vi "RLconnect.vi"() -> ()   [LabVIEW 2019]
uses:
  Ctrl/ublox-ui_main.ctl
  Ctrl/gnss_config-2.ctl
  Ctrl/Ntrip_Account_db.ctl
  Ctrl/Ntrip error-leds.ctl
  Ctrl/cmd_common.ctl
  Ctrl/cmd_ini-add-read.ctl
  Ctrl/cmd_ini-RW.ctl
  Ctrl/GNSS-Ntrip ref.ctl
  Gmap/gmap_fgv-cmd.ctl
  Ctrl/error_state-val.ctl
  Ctrl/GNSS-Ntrip config.ctl
  C:/Users/WeGo/Documents/GitHub/Ycar/LabVIEW/Gmap/dll/GMap.NET.WindowsForms.dll
  Gmap/dll/GMap.NET.WindowsForms.dll
panel:
  out "Error":T1={"GNSS Serial"=0, "NMEA val"=0, "Send Serial"=0, "Ntrip TCP"=0, "RTCM val"=0, "GMAP"=0, "TBD1"=2, "TBD2"=2, "TBD3"=2}
  in  "Send-Serial Start-Stop":bool
  in  "GNSS Start-Stop":bool
  in  "stop":bool
  in  "gmap center":bool
  in  "Gmap Lon":dbl format="%.7f"
  in  "Gmap Lat":dbl format="%.7f"
  in  "GMapControl":refnum<k24>(container)
  out "GNSS time":string
  out "Ntrip conn":bool
  out "NMEA val":bool
  in  "main tap":T2(tab)
  out "TM\nptn":u32(slide) scale=0.0..200.0
  out "Sea Level":dbl
  out "N of Satellites":i32
  out "TM graph":T3(graph)=[{"TM array"=[{"Y(E)"=195478.83340938148, "X(N)"=532749.6315443226}, {"Y(E)"=195478.83340938148, "X(N)"=532749.6315443226}, {"Y(E)"=195478.83340938148, "X(N)"=532749.6315443226}, {"Y(E)"=195478.83340938148, "X(N)"=532749.6315443226}, {"Y(E)"=195478.83340938148, "X(N)"=532749.6315443226}, {"Y(E)"=195478.83340938148, "X(N)"=532749.6315443226}, {"Y(E)"=195478.83340938148, "X(N)"=532749.6315443226}, {"Y(E)"=195478.83340938148, "X(N)"=532749.6315443226}, {"Y(E)"=195478.83340938148, "X(N)"=532749.6315443226}, {"Y(E)"=195478.83340938148, "X(N)"=532749.6315443226}, {"Y(E)"=195478.80387262133, "X(N)"=532749.5945652778}, {"Y(E)"=195478.80387262133, "X(N)"=532749.5945652778}, {"Y(E)"=195478.80387262133, "X(N)"=532749.5945652778}, {"Y(E)"=195478.80387262133, "X(N)"=532749.5945652778}, {"Y(E)"=195478.80387262133, "X(N)"=532749.5945652778}, {"Y(E)"=195478.80387262133, "X(N)"=532749.5945652778}, {"Y(E)"=195478.80387262133, "X(N)"=532749.5945652778}, {"Y(E)"=195478.80387262133, "X(N)"=532749.5945652778}, {"Y(E)"=195478.80387262133, "X(N)"=532749.5945652778}, {"Y(E)"=195478.80387262133, "X(N)"=532749.5945652778}, {"Y(E)"=195478.80387262133, "X(N)"=532749.5945652778}, {"Y(E)"=195478.80387262133, "X(N)"=532749.5945652778}, {"Y(E)"=195478.80387262133, "X(N)"=532749.5945652778}, {"Y(E)"=195478.86283602339, "X(N)"=532749.4650507653}, {"Y(E)"=195478.86283602339, "X(N)"=532749.4650507653}, {"Y(E)"=195478.86283602339, "X(N)"=532749.4650507653}, {"Y(E)"=195478.86283602339, "X(N)"=532749.4650507653}, {"Y(E)"=195478.86283602339, "X(N)"=532749.4650507653}, {"Y(E)"=195478.86283602339, "X(N)"=532749.4650507653}, {"Y(E)"=195478.86283602339, "X(N)"=532749.4650507653}, {"Y(E)"=195478.86283602339, "X(N)"=532749.4650507653}, {"Y(E)"=195478.86283602339, "X(N)"=532749.4650507653}, {"Y(E)"=195478.86283602339, "X(N)"=532749.4650507653}, {"Y(E)"=195478.86283602339, "X(N)"=532749.4650507653}, {"Y(E)"=195478.86283602339, "X(N)"=532749.4650507653}, {"Y(E)"=195478.86283602339, "X(N)"=532749.4650507653}, {"Y(E)"=195478.8185809412, "X(N)"=532749.5020697443}, {"Y(E)"=195478.8185809412, "X(N)"=532749.5020697443}, {"Y(E)"=195478.8185809412, "X(N)"=532749.5020697443}, {"Y(E)"=195478.8185809412, "X(N)"=532749.5020697443}, {"Y(E)"=195478.8185809412, "X(N)"=532749.5020697443}, {"Y(E)"=195478.8185809412, "X(N)"=532749.5020697443}, {"Y(E)"=195478.8185809412, "X(N)"=532749.5020697443}, {"Y(E)"=195478.8185809412, "X(N)"=532749.5020697443}, {"Y(E)"=195478.8185809412, "X(N)"=532749.5020697443}, {"Y(E)"=195478.8185809412, "X(N)"=532749.5020697443}, {"Y(E)"=195478.8185809412, "X(N)"=532749.5020697443}, {"Y(E)"=195478.8185809412, "X(N)"=532749.5020697443}, {"Y(E)"=195478.8185809412, "X(N)"=532749.5020697443}, {"Y(E)"=195478.8333493192, "X(N)"=532749.5205592669}, {"Y(E)"=195478.8333493192, "X(N)"=532749.5205592669}, {"Y(E)"=195478.8333493192, "X(N)"=532749.5205592669}, {"Y(E)"=195478.8333493192, "X(N)"=532749.5205592669}, {"Y(E)"=195478.8333493192, "X(N)"=532749.5205592669}, {"Y(E)"=195478.8333493192, "X(N)"=532749.5205592669}, {"Y(E)"=195478.8333493192, "X(N)"=532749.5205592669}, {"Y(E)"=195478.8333493192, "X(N)"=532749.5205592669}, {"Y(E)"=195478.8333493192, "X(N)"=532749.5205592669}, {"Y(E)"=195478.8333493192, "X(N)"=532749.5205592669}, {"Y(E)"=195478.8333493192, "X(N)"=532749.5205592669}, {"Y(E)"=195478.8333493192, "X(N)"=532749.5205592669}, {"Y(E)"=195478.81854089958, "X(N)"=532749.4280797082}, {"Y(E)"=195478.81854089958, "X(N)"=532749.4280797082}, {"Y(E)"=195478.81854089958, "X(N)"=532749.4280797082}, {"Y(E)"=195478.81854089958, "X(N)"=532749.4280797082}, {"Y(E)"=195478.81854089958, "X(N)"=532749.4280797082}, {"Y(E)"=195478.81854089958, "X(N)"=532749.4280797082}, {"Y(E)"=195478.81854089958, "X(N)"=532749.4280797082}, {"Y(E)"=195478.81854089958, "X(N)"=532749.4280797082}, {"Y(E)"=195478.81854089958, "X(N)"=532749.4280797082}, {"Y(E)"=195478.81854089958, "X(N)"=532749.4280797082}, {"Y(E)"=195478.81854089958, "X(N)"=532749.4280797082}, {"Y(E)"=195478.81854089958, "X(N)"=532749.4280797082}, {"Y(E)"=195478.81854089958, "X(N)"=532749.4280797082}, {"Y(E)"=195478.8332592258, "X(N)"=532749.3540816847}, {"Y(E)"=195478.8332592258, "X(N)"=532749.3540816847}, {"Y(E)"=195478.8332592258, "X(N)"=532749.3540816847}, {"Y(E)"=195478.8332592258, "X(N)"=532749.3540816847}, {"Y(E)"=195478.8332592258, "X(N)"=532749.3540816847}, {"Y(E)"=195478.8332592258, "X(N)"=532749.3540816847}, {"Y(E)"=195478.8332592258, "X(N)"=532749.3540816847}, {"Y(E)"=195478.8332592258, "X(N)"=532749.3540816847}, {"Y(E)"=195478.8332592258, "X(N)"=532749.3540816847}, {"Y(E)"=195478.8332592258, "X(N)"=532749.3540816847}, {"Y(E)"=195478.8332592258, "X(N)"=532749.3540816847}, {"Y(E)"=195478.8332592258, "X(N)"=532749.3540816847}, {"Y(E)"=195478.8332592258, "X(N)"=532749.3540816847}, {"Y(E)"=195478.61200383154, "X(N)"=532749.5761715989}, {"Y(E)"=195478.61200383154, "X(N)"=532749.5761715989}, {"Y(E)"=195478.61200383154, "X(N)"=532749.5761715989}, {"Y(E)"=195478.61200383154, "X(N)"=532749.5761715989}, {"Y(E)"=195478.61200383154, "X(N)"=532749.5761715989}, {"Y(E)"=195478.61200383154, "X(N)"=532749.5761715989}, {"Y(E)"=195478.61200383154, "X(N)"=532749.5761715989}, {"Y(E)"=195478.61200383154, "X(N)"=532749.5761715989}, {"Y(E)"=195478.61200383154, "X(N)"=532749.5761715989}, {"Y(E)"=195478.61200383154, "X(N)"=532749.5761715989}, {"Y(E)"=195478.61200383154, "X(N)"=532749.5761715989}, {"Y(E)"=195478.61200383154, "X(N)"=532749.5761715989}, {"Y(E)"=195478.61200383154, "X(N)"=532749.5761715989}, {"Y(E)"=195478.61197379892, "X(N)"=532749.5206790727}, {"Y(E)"=195478.61197379892, "X(N)"=532749.5206790727}, {"Y(E)"=195478.61197379892, "X(N)"=532749.5206790727}, {"Y(E)"=195478.61197379892, "X(N)"=532749.5206790727}, {"Y(E)"=195478.61197379892, "X(N)"=532749.5206790727}, {"Y(E)"=195478.61197379892, "X(N)"=532749.5206790727}, {"Y(E)"=195478.61197379892, "X(N)"=532749.5206790727}, {"Y(E)"=195478.61197379892, "X(N)"=532749.5206790727}, {"Y(E)"=195478.61197379892, "X(N)"=532749.5206790727}, {"Y(E)"=195478.61197379892, "X(N)"=532749.5206790727}, {"Y(E)"=195478.61197379892, "X(N)"=532749.5206790727}, {"Y(E)"=195478.61197379892, "X(N)"=532749.5206790727}, {"Y(E)"=195478.61197379892, "X(N)"=532749.5206790727}, {"Y(E)"=195478.64144048005, "X(N)"=532749.4281755526}, {"Y(E)"=195478.64144048005, "X(N)"=532749.4281755526}, {"Y(E)"=195478.64144048005, "X(N)"=532749.4281755526}, {"Y(E)"=195478.64144048005, "X(N)"=532749.4281755526}, {"Y(E)"=195478.64144048005, "X(N)"=532749.4281755526}, {"Y(E)"=195478.64144048005, "X(N)"=532749.4281755526}, {"Y(E)"=195478.64144048005, "X(N)"=532749.4281755526}, {"Y(E)"=195478.64144048005, "X(N)"=532749.4281755526}, {"Y(E)"=195478.64144048005, "X(N)"=532749.4281755526}, {"Y(E)"=195478.64144048005, "X(N)"=532749.4281755526}, {"Y(E)"=195478.64144048005, "X(N)"=532749.4281755526}, {"Y(E)"=195478.64144048005, "X(N)"=532749.4281755526}, {"Y(E)"=195478.64144048005, "X(N)"=532749.4281755526}, {"Y(E)"=195478.56754852948, "X(N)"=532749.2432403986}, {"Y(E)"=195478.56754852948, "X(N)"=532749.2432403986}, {"Y(E)"=195478.56754852948, "X(N)"=532749.2432403986}, {"Y(E)"=195478.56754852948, "X(N)"=532749.2432403986}, {"Y(E)"=195478.56754852948, "X(N)"=532749.2432403986}, {"Y(E)"=195478.56754852948, "X(N)"=532749.2432403986}, {"Y(E)"=195478.56754852948, "X(N)"=532749.2432403986}, {"Y(E)"=195478.56754852948, "X(N)"=532749.2432403986}, {"Y(E)"=195478.56754852948, "X(N)"=532749.2432403986}, {"Y(E)"=195478.56754852948, "X(N)"=532749.2432403986}, {"Y(E)"=195478.56754852948, "X(N)"=532749.2432403986}, {"Y(E)"=195478.56754852948, "X(N)"=532749.2432403986}, {"Y(E)"=195478.56754852948, "X(N)"=532749.2432403986}, {"Y(E)"=195478.5822568451, "X(N)"=532749.1507448669}, {"Y(E)"=195478.5822568451, "X(N)"=532749.1507448669}, {"Y(E)"=195478.5822568451, "X(N)"=532749.1507448669}, {"Y(E)"=195478.5822568451, "X(N)"=532749.1507448669}, {"Y(E)"=195478.5822568451, "X(N)"=532749.1507448669}, {"Y(E)"=195478.5822568451, "X(N)"=532749.1507448669}, {"Y(E)"=195478.5822568451, "X(N)"=532749.1507448669}, {"Y(E)"=195478.5822568451, "X(N)"=532749.1507448669}, {"Y(E)"=195478.5822568451, "X(N)"=532749.1507448669}, {"Y(E)"=195478.5822568451, "X(N)"=532749.1507448669}, {"Y(E)"=195478.5822568451, "X(N)"=532749.1507448669}, {"Y(E)"=195478.5822568451, "X(N)"=532749.1507448669}, {"Y(E)"=195478.5822568451, "X(N)"=532749.1507448669}, {"Y(E)"=195478.3755095352, "X(N)"=532748.9103890732}, {"Y(E)"=195478.3755095352, "X(N)"=532748.9103890732}, {"Y(E)"=195478.3755095352, "X(N)"=532748.9103890732}, {"Y(E)"=195478.3755095352, "X(N)"=532748.9103890732}, {"Y(E)"=195478.3755095352, "X(N)"=532748.9103890732}, {"Y(E)"=195478.3755095352, "X(N)"=532748.9103890732}, {"Y(E)"=195478.3755095352, "X(N)"=532748.9103890732}, {"Y(E)"=195478.3755095352, "X(N)"=532748.9103890732}, {"Y(E)"=195478.3755095352, "X(N)"=532748.9103890732}, {"Y(E)"=195478.3755095352, "X(N)"=532748.9103890732}, {"Y(E)"=195478.3755095352, "X(N)"=532748.9103890732}, {"Y(E)"=195478.3755095352, "X(N)"=532748.9103890732}, {"Y(E)"=195478.3755095352, "X(N)"=532748.9103890732}, {"Y(E)"=195478.37543945547, "X(N)"=532748.78090651}, {"Y(E)"=195478.37543945547, "X(N)"=532748.78090651}, {"Y(E)"=195478.37543945547, "X(N)"=532748.78090651}, {"Y(E)"=195478.37543945547, "X(N)"=532748.78090651}, {"Y(E)"=195478.37543945547, "X(N)"=532748.78090651}, {"Y(E)"=195478.37543945547, "X(N)"=532748.78090651}, {"Y(E)"=195478.37543945547, "X(N)"=532748.78090651}, {"Y(E)"=195478.37543945547, "X(N)"=532748.78090651}, {"Y(E)"=195478.37543945547, "X(N)"=532748.78090651}, {"Y(E)"=195478.37543945547, "X(N)"=532748.78090651}, {"Y(E)"=195478.37543945547, "X(N)"=532748.78090651}, {"Y(E)"=195478.37543945547, "X(N)"=532748.78090651}, {"Y(E)"=195478.5082848043, "X(N)"=532748.8178296402}, {"Y(E)"=195478.5082848043, "X(N)"=532748.8178296402}, {"Y(E)"=195478.5082848043, "X(N)"=532748.8178296402}, {"Y(E)"=195478.5082848043, "X(N)"=532748.8178296402}, {"Y(E)"=195478.5082848043, "X(N)"=532748.8178296402}, {"Y(E)"=195478.5082848043, "X(N)"=532748.8178296402}, {"Y(E)"=195478.5082848043, "X(N)"=532748.8178296402}, {"Y(E)"=195478.5082848043, "X(N)"=532748.8178296402}, {"Y(E)"=195478.5082848043, "X(N)"=532748.8178296402}, {"Y(E)"=195478.5082848043, "X(N)"=532748.8178296402}, {"Y(E)"=195478.5082848043, "X(N)"=532748.8178296402}, {"Y(E)"=195478.5082848043, "X(N)"=532748.8178296402}, {"Y(E)"=195478.5082848043, "X(N)"=532748.8178296402}, {"Y(E)"=195478.7001636224, "X(N)"=532748.8547208244}, {"Y(E)"=195478.7001636224, "X(N)"=532748.8547208244}, {"Y(E)"=195478.7001636224, "X(N)"=532748.8547208244}, {"Y(E)"=195478.7001636224, "X(N)"=532748.8547208244}, {"Y(E)"=195478.7001636224, "X(N)"=532748.8547208244}, {"Y(E)"=195478.7001636224, "X(N)"=532748.8547208244}, {"Y(E)"=195478.7001636224, "X(N)"=532748.8547208244}, {"Y(E)"=195478.7001636224, "X(N)"=532748.8547208244}, {"Y(E)"=195478.7001636224, "X(N)"=532748.8547208244}, {"Y(E)"=195478.7001636224, "X(N)"=532748.8547208244}]}, {"TM array"=[{"Y(E)"=195478.60442441847, "X(N)"=532749.6892681528}, {"Y(E)"=195478.63475492285, "X(N)"=532749.6883149784}, {"Y(E)"=195478.6649657266, "X(N)"=532749.6854592166}, {"Y(E)"=195478.69493760145, "X(N)"=532749.680712138}, {"Y(E)"=195478.72455226214, "X(N)"=532749.6740924771}, {"Y(E)"=195478.7536928331, "X(N)"=532749.6656263586}, {"Y(E)"=195478.7822443098, "X(N)"=532749.6553471944}, {"Y(E)"=195478.81009401265, "X(N)"=532749.6432955518}, {"Y(E)"=195478.83713203156, "X(N)"=532749.6295189931}, {"Y(E)"=195478.86325165984, "X(N)"=532749.6140718879}, {"Y(E)"=195478.88834981524, "X(N)"=532749.5970151991}, {"Y(E)"=195478.91232744683, "X(N)"=532749.5784162417}, {"Y(E)"=195478.93508992583, "X(N)"=532749.5583484169}, {"Y(E)"=195478.95654741913, "X(N)"=532749.5368909236}, {"Y(E)"=195478.97661524382, "X(N)"=532749.5141284446}, {"Y(E)"=195478.99521420136, "X(N)"=532749.490150813}, {"Y(E)"=195479.01227089018, "X(N)"=532749.4650526576}, {"Y(E)"=195479.02771799528, "X(N)"=532749.4389330294}, {"Y(E)"=195479.04149455403, "X(N)"=532749.4118950105}, {"Y(E)"=195479.0535461966, "X(N)"=532749.3840453076}, {"Y(E)"=195479.06382536073, "X(N)"=532749.3554938309}, {"Y(E)"=195479.0722914792, "X(N)"=532749.32635326}, {"Y(E)"=195479.07891114015, "X(N)"=532749.2967385993}, {"Y(E)"=195479.0836582188, "X(N)"=532749.2667667244}, {"Y(E)"=195479.08651398055, "X(N)"=532749.2365559207}, {"Y(E)"=195479.08746715504, "X(N)"=532749.2062254163}, {"Y(E)"=195479.08651398055, "X(N)"=532749.1758949119}, {"Y(E)"=195479.0836582188, "X(N)"=532749.1456841081}, {"Y(E)"=195479.07891114015, "X(N)"=532749.1157122332}, {"Y(E)"=195479.0722914792, "X(N)"=532749.0860975726}, {"Y(E)"=195479.06382536073, "X(N)"=532749.0569570017}, {"Y(E)"=195479.0535461966, "X(N)"=532749.0284055249}, {"Y(E)"=195479.04149455403, "X(N)"=532749.000555822}, {"Y(E)"=195479.02771799528, "X(N)"=532748.9735178031}, {"Y(E)"=195479.01227089018, "X(N)"=532748.9473981749}, {"Y(E)"=195478.99521420136, "X(N)"=532748.9223000195}, {"Y(E)"=195478.97661524382, "X(N)"=532748.898322388}, {"Y(E)"=195478.95654741913, "X(N)"=532748.8755599089}, {"Y(E)"=195478.93508992583, "X(N)"=532748.8541024156}, {"Y(E)"=195478.91232744683, "X(N)"=532748.8340345909}, {"Y(E)"=195478.88834981524, "X(N)"=532748.8154356334}, {"Y(E)"=195478.86325165984, "X(N)"=532748.7983789446}, {"Y(E)"=195478.83713203156, "X(N)"=532748.7829318395}, {"Y(E)"=195478.81009401265, "X(N)"=532748.7691552808}, {"Y(E)"=195478.7822443098, "X(N)"=532748.7571036381}, {"Y(E)"=195478.7536928331, "X(N)"=532748.746824474}, {"Y(E)"=195478.72455226214, "X(N)"=532748.7383583555}, {"Y(E)"=195478.69493760145, "X(N)"=532748.7317386946}, {"Y(E)"=195478.6649657266, "X(N)"=532748.726991616}, {"Y(E)"=195478.63475492285, "X(N)"=532748.7241358542}, {"Y(E)"=195478.60442441847, "X(N)"=532748.7231826797}, {"Y(E)"=195478.5740939141, "X(N)"=532748.7241358542}, {"Y(E)"=195478.54388311034, "X(N)"=532748.726991616}, {"Y(E)"=195478.5139112355, "X(N)"=532748.7317386946}, {"Y(E)"=195478.4842965748, "X(N)"=532748.7383583555}, {"Y(E)"=195478.45515600385, "X(N)"=532748.746824474}, {"Y(E)"=195478.42660452714, "X(N)"=532748.7571036381}, {"Y(E)"=195478.3987548243, "X(N)"=532748.7691552808}, {"Y(E)"=195478.37171680538, "X(N)"=532748.7829318395}, {"Y(E)"=195478.3455971771, "X(N)"=532748.7983789446}, {"Y(E)"=195478.3204990217, "X(N)"=532748.8154356334}, {"Y(E)"=195478.29652139012, "X(N)"=532748.8340345909}, {"Y(E)"=195478.27375891112, "X(N)"=532748.8541024156}, {"Y(E)"=195478.25230141782, "X(N)"=532748.8755599089}, {"Y(E)"=195478.23223359312, "X(N)"=532748.898322388}, {"Y(E)"=195478.21363463558, "X(N)"=532748.9223000195}, {"Y(E)"=195478.19657794677, "X(N)"=532748.9473981749}, {"Y(E)"=195478.18113084167, "X(N)"=532748.9735178031}, {"Y(E)"=195478.16735428292, "X(N)"=532749.000555822}, {"Y(E)"=195478.15530264034, "X(N)"=532749.0284055249}, {"Y(E)"=195478.14502347622, "X(N)"=532749.0569570017}, {"Y(E)"=195478.13655735774, "X(N)"=532749.0860975726}, {"Y(E)"=195478.1299376968, "X(N)"=532749.1157122332}, {"Y(E)"=195478.12519061816, "X(N)"=532749.1456841081}, {"Y(E)"=195478.1223348564, "X(N)"=532749.1758949119}, {"Y(E)"=195478.1213816819, "X(N)"=532749.2062254163}, {"Y(E)"=195478.1223348564, "X(N)"=532749.2365559207}, {"Y(E)"=195478.12519061816, "X(N)"=532749.2667667244}, {"Y(E)"=195478.1299376968, "X(N)"=532749.2967385993}, {"Y(E)"=195478.13655735774, "X(N)"=532749.32635326}, {"Y(E)"=195478.14502347622, "X(N)"=532749.3554938309}, {"Y(E)"=195478.15530264034, "X(N)"=532749.3840453076}, {"Y(E)"=195478.16735428292, "X(N)"=532749.4118950105}, {"Y(E)"=195478.18113084167, "X(N)"=532749.4389330294}, {"Y(E)"=195478.19657794677, "X(N)"=532749.4650526576}, {"Y(E)"=195478.21363463558, "X(N)"=532749.490150813}, {"Y(E)"=195478.23223359312, "X(N)"=532749.5141284446}, {"Y(E)"=195478.25230141782, "X(N)"=532749.5368909236}, {"Y(E)"=195478.27375891112, "X(N)"=532749.5583484169}, {"Y(E)"=195478.29652139012, "X(N)"=532749.5784162417}, {"Y(E)"=195478.3204990217, "X(N)"=532749.5970151991}, {"Y(E)"=195478.3455971771, "X(N)"=532749.6140718879}, {"Y(E)"=195478.37171680538, "X(N)"=532749.6295189931}, {"Y(E)"=195478.3987548243, "X(N)"=532749.6432955518}, {"Y(E)"=195478.42660452714, "X(N)"=532749.6553471944}, {"Y(E)"=195478.45515600385, "X(N)"=532749.6656263586}, {"Y(E)"=195478.4842965748, "X(N)"=532749.6740924771}, {"Y(E)"=195478.5139112355, "X(N)"=532749.680712138}, {"Y(E)"=195478.54388311034, "X(N)"=532749.6854592166}, {"Y(E)"=195478.5740939141, "X(N)"=532749.6883149784}, {"Y(E)"=195478.60442441847, "X(N)"=532749.6892681528}]}, {"TM array"=[{"Y(E)"=195478.60442441847, "X(N)"=532750.2062254163}, {"Y(E)"=195478.667214938, "X(N)"=532750.2042521447}, {"Y(E)"=195478.72975765204, "X(N)"=532750.1983401176}, {"Y(E)"=195478.79180573305, "X(N)"=532750.188512667}, {"Y(E)"=195478.85311430565, "X(N)"=532750.1748085774}, {"Y(E)"=195478.91344141285, "X(N)"=532750.1572819325}, {"Y(E)"=195478.97254897116, "X(N)"=532750.1360019022}, {"Y(E)"=195479.03020371005, "X(N)"=532750.1110524688}, {"Y(E)"=195479.08617809258, "X(N)"=532750.0825320963}, {"Y(E)"=195479.14025121345, "X(N)"=532750.0505533417}, {"Y(E)"=195479.19220967076, "X(N)"=532750.0152424106}, {"Y(E)"=195479.24184840822, "X(N)"=532749.9767386591}, {"Y(E)"=195479.2889715244, "X(N)"=532749.9351940437}, {"Y(E)"=195479.3333930459, "X(N)"=532749.8907725222}, {"Y(E)"=195479.37493766125, "X(N)"=532749.843649406}, {"Y(E)"=195479.41344141285, "X(N)"=532749.7940106685}, {"Y(E)"=195479.44875234397, "X(N)"=532749.7420522113}, {"Y(E)"=195479.4807310985, "X(N)"=532749.6879790904}, {"Y(E)"=195479.50925147094, "X(N)"=532749.6320047078}, {"Y(E)"=195479.53420090437, "X(N)"=532749.5743499689}, {"Y(E)"=195479.55548093477, "X(N)"=532749.5152424106}, {"Y(E)"=195479.5730075796, "X(N)"=532749.4549153034}, {"Y(E)"=195479.5867116692, "X(N)"=532749.3936067309}, {"Y(E)"=195479.59653911978, "X(N)"=532749.3315586499}, {"Y(E)"=195479.6024511469, "X(N)"=532749.2690159358}, {"Y(E)"=195479.60442441847, "X(N)"=532749.2062254163}, {"Y(E)"=195479.6024511469, "X(N)"=532749.1434348967}, {"Y(E)"=195479.59653911978, "X(N)"=532749.0808921827}, {"Y(E)"=195479.5867116692, "X(N)"=532749.0188441017}, {"Y(E)"=195479.5730075796, "X(N)"=532748.9575355292}, {"Y(E)"=195479.55548093477, "X(N)"=532748.897208422}, {"Y(E)"=195479.53420090437, "X(N)"=532748.8381008636}, {"Y(E)"=195479.50925147094, "X(N)"=532748.7804461247}, {"Y(E)"=195479.4807310985, "X(N)"=532748.7244717422}, {"Y(E)"=195479.44875234397, "X(N)"=532748.6703986212}, {"Y(E)"=195479.41344141285, "X(N)"=532748.618440164}, {"Y(E)"=195479.37493766125, "X(N)"=532748.5688014266}, {"Y(E)"=195479.3333930459, "X(N)"=532748.5216783104}, {"Y(E)"=195479.2889715244, "X(N)"=532748.4772567889}, {"Y(E)"=195479.24184840822, "X(N)"=532748.4357121735}, {"Y(E)"=195479.19220967076, "X(N)"=532748.397208422}, {"Y(E)"=195479.14025121345, "X(N)"=532748.3618974908}, {"Y(E)"=195479.08617809258, "X(N)"=532748.3299187362}, {"Y(E)"=195479.03020371005, "X(N)"=532748.3013983638}, {"Y(E)"=195478.97254897116, "X(N)"=532748.2764489304}, {"Y(E)"=195478.91344141285, "X(N)"=532748.2551689}, {"Y(E)"=195478.85311430565, "X(N)"=532748.2376422551}, {"Y(E)"=195478.79180573305, "X(N)"=532748.2239381656}, {"Y(E)"=195478.72975765204, "X(N)"=532748.214110715}, {"Y(E)"=195478.667214938, "X(N)"=532748.2081986879}, {"Y(E)"=195478.60442441847, "X(N)"=532748.2062254163}, {"Y(E)"=195478.54163389895, "X(N)"=532748.2081986879}, {"Y(E)"=195478.4790911849, "X(N)"=532748.214110715}, {"Y(E)"=195478.4170431039, "X(N)"=532748.2239381656}, {"Y(E)"=195478.3557345313, "X(N)"=532748.2376422551}, {"Y(E)"=195478.2954074241, "X(N)"=532748.2551689}, {"Y(E)"=195478.2362998658, "X(N)"=532748.2764489304}, {"Y(E)"=195478.1786451269, "X(N)"=532748.3013983638}, {"Y(E)"=195478.12267074437, "X(N)"=532748.3299187362}, {"Y(E)"=195478.0685976235, "X(N)"=532748.3618974908}, {"Y(E)"=195478.0166391662, "X(N)"=532748.397208422}, {"Y(E)"=195477.96700042873, "X(N)"=532748.4357121735}, {"Y(E)"=195477.91987731255, "X(N)"=532748.4772567889}, {"Y(E)"=195477.87545579104, "X(N)"=532748.5216783104}, {"Y(E)"=195477.8339111757, "X(N)"=532748.5688014266}, {"Y(E)"=195477.7954074241, "X(N)"=532748.618440164}, {"Y(E)"=195477.76009649297, "X(N)"=532748.6703986212}, {"Y(E)"=195477.72811773844, "X(N)"=532748.7244717422}, {"Y(E)"=195477.699597366, "X(N)"=532748.7804461247}, {"Y(E)"=195477.67464793258, "X(N)"=532748.8381008636}, {"Y(E)"=195477.65336790218, "X(N)"=532748.897208422}, {"Y(E)"=195477.63584125735, "X(N)"=532748.9575355292}, {"Y(E)"=195477.62213716775, "X(N)"=532749.0188441017}, {"Y(E)"=195477.61230971717, "X(N)"=532749.0808921827}, {"Y(E)"=195477.60639769005, "X(N)"=532749.1434348967}, {"Y(E)"=195477.60442441847, "X(N)"=532749.2062254163}, {"Y(E)"=195477.60639769005, "X(N)"=532749.2690159358}, {"Y(E)"=195477.61230971717, "X(N)"=532749.3315586499}, {"Y(E)"=195477.62213716775, "X(N)"=532749.3936067309}, {"Y(E)"=195477.63584125735, "X(N)"=532749.4549153034}, {"Y(E)"=195477.65336790218, "X(N)"=532749.5152424106}, {"Y(E)"=195477.67464793258, "X(N)"=532749.5743499689}, {"Y(E)"=195477.699597366, "X(N)"=532749.6320047078}, {"Y(E)"=195477.72811773844, "X(N)"=532749.6879790904}, {"Y(E)"=195477.76009649297, "X(N)"=532749.7420522113}, {"Y(E)"=195477.7954074241, "X(N)"=532749.7940106685}, {"Y(E)"=195477.8339111757, "X(N)"=532749.843649406}, {"Y(E)"=195477.87545579104, "X(N)"=532749.8907725222}, {"Y(E)"=195477.91987731255, "X(N)"=532749.9351940437}, {"Y(E)"=195477.96700042873, "X(N)"=532749.9767386591}, {"Y(E)"=195478.0166391662, "X(N)"=532750.0152424106}, {"Y(E)"=195478.0685976235, "X(N)"=532750.0505533417}, {"Y(E)"=195478.12267074437, "X(N)"=532750.0825320963}, {"Y(E)"=195478.1786451269, "X(N)"=532750.1110524688}, {"Y(E)"=195478.2362998658, "X(N)"=532750.1360019022}, {"Y(E)"=195478.2954074241, "X(N)"=532750.1572819325}, {"Y(E)"=195478.3557345313, "X(N)"=532750.1748085774}, {"Y(E)"=195478.4170431039, "X(N)"=532750.188512667}, {"Y(E)"=195478.4790911849, "X(N)"=532750.1983401176}, {"Y(E)"=195478.54163389895, "X(N)"=532750.2042521447}, {"Y(E)"=195478.60442441847, "X(N)"=532750.2062254163}]}, {"TM array"=[{"Y(E)"=195478.60442441847, "X(N)"=532751.2062254163}, {"Y(E)"=195478.73000545753, "X(N)"=532751.2022788732}, {"Y(E)"=195478.8550908856, "X(N)"=532751.1904548189}, {"Y(E)"=195478.97918704763, "X(N)"=532751.1707999178}, {"Y(E)"=195479.10180419282, "X(N)"=532751.1433917385}, {"Y(E)"=195479.22245840722, "X(N)"=532751.1083384489}, {"Y(E)"=195479.34067352384, "X(N)"=532751.0657783881}, {"Y(E)"=195479.4559830016, "X(N)"=532751.0158795213}, {"Y(E)"=195479.56793176668, "X(N)"=532750.9588387763}, {"Y(E)"=195479.67607800843, "X(N)"=532750.8948812673}, {"Y(E)"=195479.77999492307, "X(N)"=532750.824259405}, {"Y(E)"=195479.879272398, "X(N)"=532750.7472519018}, {"Y(E)"=195479.97351863034, "X(N)"=532750.6641626711}, {"Y(E)"=195480.0623616733, "X(N)"=532750.5753196281}, {"Y(E)"=195480.14545090403, "X(N)"=532750.4810733958}, {"Y(E)"=195480.22245840722, "X(N)"=532750.3817959209}, {"Y(E)"=195480.29308026948, "X(N)"=532750.2778790062}, {"Y(E)"=195480.35703777857, "X(N)"=532750.1697327645}, {"Y(E)"=195480.4140785234, "X(N)"=532750.0577839994}, {"Y(E)"=195480.46397739026, "X(N)"=532749.9424745217}, {"Y(E)"=195480.50653745106, "X(N)"=532749.824259405}, {"Y(E)"=195480.54159074073, "X(N)"=532749.7036051906}, {"Y(E)"=195480.56899891995, "X(N)"=532749.5809880454}, {"Y(E)"=195480.5886538211, "X(N)"=532749.4568918834}, {"Y(E)"=195480.60047787533, "X(N)"=532749.3318064554}, {"Y(E)"=195480.60442441847, "X(N)"=532749.2062254163}, {"Y(E)"=195480.60047787533, "X(N)"=532749.0806443772}, {"Y(E)"=195480.5886538211, "X(N)"=532748.9555589492}, {"Y(E)"=195480.56899891995, "X(N)"=532748.8314627871}, {"Y(E)"=195480.54159074073, "X(N)"=532748.7088456419}, {"Y(E)"=195480.50653745106, "X(N)"=532748.5881914275}, {"Y(E)"=195480.46397739026, "X(N)"=532748.4699763109}, {"Y(E)"=195480.4140785234, "X(N)"=532748.3546668332}, {"Y(E)"=195480.35703777857, "X(N)"=532748.2427180681}, {"Y(E)"=195480.29308026948, "X(N)"=532748.1345718263}, {"Y(E)"=195480.22245840722, "X(N)"=532748.0306549117}, {"Y(E)"=195480.14545090403, "X(N)"=532747.9313774367}, {"Y(E)"=195480.0623616733, "X(N)"=532747.8371312044}, {"Y(E)"=195479.97351863034, "X(N)"=532747.7482881615}, {"Y(E)"=195479.879272398, "X(N)"=532747.6651989308}, {"Y(E)"=195479.77999492307, "X(N)"=532747.5881914275}, {"Y(E)"=195479.67607800843, "X(N)"=532747.5175695652}, {"Y(E)"=195479.56793176668, "X(N)"=532747.4536120562}, {"Y(E)"=195479.4559830016, "X(N)"=532747.3965713113}, {"Y(E)"=195479.34067352384, "X(N)"=532747.3466724445}, {"Y(E)"=195479.22245840722, "X(N)"=532747.3041123836}, {"Y(E)"=195479.10180419282, "X(N)"=532747.269059094}, {"Y(E)"=195478.97918704763, "X(N)"=532747.2416509148}, {"Y(E)"=195478.8550908856, "X(N)"=532747.2219960137}, {"Y(E)"=195478.73000545753, "X(N)"=532747.2101719594}, {"Y(E)"=195478.60442441847, "X(N)"=532747.2062254163}, {"Y(E)"=195478.47884337942, "X(N)"=532747.2101719594}, {"Y(E)"=195478.35375795135, "X(N)"=532747.2219960137}, {"Y(E)"=195478.22966178932, "X(N)"=532747.2416509148}, {"Y(E)"=195478.10704464413, "X(N)"=532747.269059094}, {"Y(E)"=195477.98639042972, "X(N)"=532747.3041123836}, {"Y(E)"=195477.8681753131, "X(N)"=532747.3466724445}, {"Y(E)"=195477.75286583535, "X(N)"=532747.3965713113}, {"Y(E)"=195477.64091707027, "X(N)"=532747.4536120562}, {"Y(E)"=195477.53277082852, "X(N)"=532747.5175695652}, {"Y(E)"=195477.42885391388, "X(N)"=532747.5881914275}, {"Y(E)"=195477.32957643896, "X(N)"=532747.6651989308}, {"Y(E)"=195477.2353302066, "X(N)"=532747.7482881615}, {"Y(E)"=195477.14648716364, "X(N)"=532747.8371312044}, {"Y(E)"=195477.0633979329, "X(N)"=532747.9313774367}, {"Y(E)"=195476.98639042972, "X(N)"=532748.0306549117}, {"Y(E)"=195476.91576856747, "X(N)"=532748.1345718263}, {"Y(E)"=195476.85181105838, "X(N)"=532748.2427180681}, {"Y(E)"=195476.79477031354, "X(N)"=532748.3546668332}, {"Y(E)"=195476.7448714467, "X(N)"=532748.4699763109}, {"Y(E)"=195476.7023113859, "X(N)"=532748.5881914275}, {"Y(E)"=195476.66725809622, "X(N)"=532748.7088456419}, {"Y(E)"=195476.639849917, "X(N)"=532748.8314627871}, {"Y(E)"=195476.62019501586, "X(N)"=532748.9555589492}, {"Y(E)"=195476.60837096162, "X(N)"=532749.0806443772}, {"Y(E)"=195476.60442441847, "X(N)"=532749.2062254163}, {"Y(E)"=195476.60837096162, "X(N)"=532749.3318064554}, {"Y(E)"=195476.62019501586, "X(N)"=532749.4568918834}, {"Y(E)"=195476.639849917, "X(N)"=532749.5809880454}, {"Y(E)"=195476.66725809622, "X(N)"=532749.7036051906}, {"Y(E)"=195476.7023113859, "X(N)"=532749.824259405}, {"Y(E)"=195476.7448714467, "X(N)"=532749.9424745217}, {"Y(E)"=195476.79477031354, "X(N)"=532750.0577839994}, {"Y(E)"=195476.85181105838, "X(N)"=532750.1697327645}, {"Y(E)"=195476.91576856747, "X(N)"=532750.2778790062}, {"Y(E)"=195476.98639042972, "X(N)"=532750.3817959209}, {"Y(E)"=195477.0633979329, "X(N)"=532750.4810733958}, {"Y(E)"=195477.14648716364, "X(N)"=532750.5753196281}, {"Y(E)"=195477.2353302066, "X(N)"=532750.6641626711}, {"Y(E)"=195477.32957643896, "X(N)"=532750.7472519018}, {"Y(E)"=195477.42885391388, "X(N)"=532750.824259405}, {"Y(E)"=195477.53277082852, "X(N)"=532750.8948812673}, {"Y(E)"=195477.64091707027, "X(N)"=532750.9588387763}, {"Y(E)"=195477.75286583535, "X(N)"=532751.0158795213}, {"Y(E)"=195477.8681753131, "X(N)"=532751.0657783881}, {"Y(E)"=195477.98639042972, "X(N)"=532751.1083384489}, {"Y(E)"=195478.10704464413, "X(N)"=532751.1433917385}, {"Y(E)"=195478.22966178932, "X(N)"=532751.1707999178}, {"Y(E)"=195478.35375795135, "X(N)"=532751.1904548189}, {"Y(E)"=195478.47884337942, "X(N)"=532751.2022788732}, {"Y(E)"=195478.60442441847, "X(N)"=532751.2062254163}]}, {"TM array"=[{"Y(E)"=195478.60442441847, "X(N)"=532752.2062254163}, {"Y(E)"=195478.79279597706, "X(N)"=532752.2003056016}, {"Y(E)"=195478.98042411916, "X(N)"=532752.1825695202}, {"Y(E)"=195479.16656836224, "X(N)"=532752.1530871685}, {"Y(E)"=195479.35049407996, "X(N)"=532752.1119748997}, {"Y(E)"=195479.5314754016, "X(N)"=532752.0593949652}, {"Y(E)"=195479.70879807652, "X(N)"=532751.995554874}, {"Y(E)"=195479.88176229317, "X(N)"=532751.9207065736}, {"Y(E)"=195480.04968544078, "X(N)"=532751.8351454564}, {"Y(E)"=195480.2119048034, "X(N)"=532751.7392091928}, {"Y(E)"=195480.36778017535, "X(N)"=532751.6332763993}, {"Y(E)"=195480.51669638773, "X(N)"=532751.5177651446}, {"Y(E)"=195480.65806573626, "X(N)"=532751.3931312986}, {"Y(E)"=195480.79133030074, "X(N)"=532751.259866734}, {"Y(E)"=195480.9159641468, "X(N)"=532751.1184973855}, {"Y(E)"=195481.0314754016, "X(N)"=532750.9695811732}, {"Y(E)"=195481.13740819498, "X(N)"=532750.8137058013}, {"Y(E)"=195481.2333444586, "X(N)"=532750.6514864386}, {"Y(E)"=195481.31890557587, "X(N)"=532750.483563291}, {"Y(E)"=195481.39375387615, "X(N)"=532750.3105990743}, {"Y(E)"=195481.45759396735, "X(N)"=532750.1332763993}, {"Y(E)"=195481.51017390186, "X(N)"=532749.9522950777}, {"Y(E)"=195481.55128617067, "X(N)"=532749.76836936}, {"Y(E)"=195481.58076852243, "X(N)"=532749.582225117}, {"Y(E)"=195481.59850460375, "X(N)"=532749.3945969748}, {"Y(E)"=195481.60442441847, "X(N)"=532749.2062254163}, {"Y(E)"=195481.59850460375, "X(N)"=532749.0178538577}, {"Y(E)"=195481.58076852243, "X(N)"=532748.8302257155}, {"Y(E)"=195481.55128617067, "X(N)"=532748.6440814725}, {"Y(E)"=195481.51017390186, "X(N)"=532748.4601557548}, {"Y(E)"=195481.45759396735, "X(N)"=532748.2791744332}, {"Y(E)"=195481.39375387615, "X(N)"=532748.1018517582}, {"Y(E)"=195481.31890557587, "X(N)"=532747.9288875415}, {"Y(E)"=195481.2333444586, "X(N)"=532747.760964394}, {"Y(E)"=195481.13740819498, "X(N)"=532747.5987450313}, {"Y(E)"=195481.0314754016, "X(N)"=532747.4428696594}, {"Y(E)"=195480.9159641468, "X(N)"=532747.293953447}, {"Y(E)"=195480.79133030074, "X(N)"=532747.1525840985}, {"Y(E)"=195480.65806573626, "X(N)"=532747.019319534}, {"Y(E)"=195480.51669638773, "X(N)"=532746.894685688}, {"Y(E)"=195480.36778017535, "X(N)"=532746.7791744332}, {"Y(E)"=195480.2119048034, "X(N)"=532746.6732416397}, {"Y(E)"=195480.04968544078, "X(N)"=532746.5773053762}, {"Y(E)"=195479.88176229317, "X(N)"=532746.4917442589}, {"Y(E)"=195479.70879807652, "X(N)"=532746.4168959586}, {"Y(E)"=195479.5314754016, "X(N)"=532746.3530558674}, {"Y(E)"=195479.35049407996, "X(N)"=532746.3004759329}, {"Y(E)"=195479.16656836224, "X(N)"=532746.2593636641}, {"Y(E)"=195478.98042411916, "X(N)"=532746.2298813123}, {"Y(E)"=195478.79279597706, "X(N)"=532746.212145231}, {"Y(E)"=195478.60442441847, "X(N)"=532746.2062254163}, {"Y(E)"=195478.4160528599, "X(N)"=532746.212145231}, {"Y(E)"=195478.2284247178, "X(N)"=532746.2298813123}, {"Y(E)"=195478.0422804747, "X(N)"=532746.2593636641}, {"Y(E)"=195477.858354757, "X(N)"=532746.3004759329}, {"Y(E)"=195477.67737343535, "X(N)"=532746.3530558674}, {"Y(E)"=195477.50005076043, "X(N)"=532746.4168959586}, {"Y(E)"=195477.32708654378, "X(N)"=532746.4917442589}, {"Y(E)"=195477.15916339617, "X(N)"=532746.5773053762}, {"Y(E)"=195476.99694403354, "X(N)"=532746.6732416397}, {"Y(E)"=195476.8410686616, "X(N)"=532746.7791744332}, {"Y(E)"=195476.69215244922, "X(N)"=532746.894685688}, {"Y(E)"=195476.55078310068, "X(N)"=532747.019319534}, {"Y(E)"=195476.4175185362, "X(N)"=532747.1525840985}, {"Y(E)"=195476.29288469013, "X(N)"=532747.293953447}, {"Y(E)"=195476.17737343535, "X(N)"=532747.4428696594}, {"Y(E)"=195476.07144064197, "X(N)"=532747.5987450313}, {"Y(E)"=195475.97550437835, "X(N)"=532747.760964394}, {"Y(E)"=195475.88994326108, "X(N)"=532747.9288875415}, {"Y(E)"=195475.8150949608, "X(N)"=532748.1018517582}, {"Y(E)"=195475.7512548696, "X(N)"=532748.2791744332}, {"Y(E)"=195475.6986749351, "X(N)"=532748.4601557548}, {"Y(E)"=195475.65756266628, "X(N)"=532748.6440814725}, {"Y(E)"=195475.62808031452, "X(N)"=532748.8302257155}, {"Y(E)"=195475.6103442332, "X(N)"=532749.0178538577}, {"Y(E)"=195475.60442441847, "X(N)"=532749.2062254163}, {"Y(E)"=195475.6103442332, "X(N)"=532749.3945969748}, {"Y(E)"=195475.62808031452, "X(N)"=532749.582225117}, {"Y(E)"=195475.65756266628, "X(N)"=532749.76836936}, {"Y(E)"=195475.6986749351, "X(N)"=532749.9522950777}, {"Y(E)"=195475.7512548696, "X(N)"=532750.1332763993}, {"Y(E)"=195475.8150949608, "X(N)"=532750.3105990743}, {"Y(E)"=195475.88994326108, "X(N)"=532750.483563291}, {"Y(E)"=195475.97550437835, "X(N)"=532750.6514864386}, {"Y(E)"=195476.07144064197, "X(N)"=532750.8137058013}, {"Y(E)"=195476.17737343535, "X(N)"=532750.9695811732}, {"Y(E)"=195476.29288469013, "X(N)"=532751.1184973855}, {"Y(E)"=195476.4175185362, "X(N)"=532751.259866734}, {"Y(E)"=195476.55078310068, "X(N)"=532751.3931312986}, {"Y(E)"=195476.69215244922, "X(N)"=532751.5177651446}, {"Y(E)"=195476.8410686616, "X(N)"=532751.6332763993}, {"Y(E)"=195476.99694403354, "X(N)"=532751.7392091928}, {"Y(E)"=195477.15916339617, "X(N)"=532751.8351454564}, {"Y(E)"=195477.32708654378, "X(N)"=532751.9207065736}, {"Y(E)"=195477.50005076043, "X(N)"=532751.995554874}, {"Y(E)"=195477.67737343535, "X(N)"=532752.0593949652}, {"Y(E)"=195477.858354757, "X(N)"=532752.1119748997}, {"Y(E)"=195478.0422804747, "X(N)"=532752.1530871685}, {"Y(E)"=195478.2284247178, "X(N)"=532752.1825695202}, {"Y(E)"=195478.4160528599, "X(N)"=532752.2003056016}, {"Y(E)"=195478.60442441847, "X(N)"=532752.2062254163}]}]
  out "GNSS data info":T4 {"HDOP" scale=0.0..10.0; "PDOP" scale=0.0..10.0; "2D Acc.m" scale=0.0..10.0; "Latitude" format="%.9f"; "Longitude" format="%.9f"; "3D Acc.m" scale=0.0..10.0}
  in  "gnss tm config":T5(tab)
  out "gnss mode cnt":u32[](array[numeric])
  out "Histogram Graph":cluster{i32[], dbl[]}(graph)
  in  "gnss mode check":bool
  out "Min circle R":dbl format="%.2g"
  out "Points size":i32
  out "loop count":i32
  in  "tm data reset":bool
  in  "TMarr-size limit":i32=200
  in  "Ref r size":dbl=1.0 format="%.2f"
  in  "Auto\ncenter":bool
  in  "PinDropMrkr":T6(ring)=enum."red_dot" caption="Pin Drop Marker"
  out "xcenter_TM":dbl
  out "ycenter_TM":dbl
  in  "Lat Dbclk":dbl format="%.11f"
  in  "Lon Dbclk":dbl format="%.11f"
  in  "Center \nupdate s":i32=10000
  in  "zoom":dbl(slide) scale=3.0..20.0
  out "NMEA cluster":T7
  out "Sel NMEA":string
  in  "Sel NMEA type":T8(ring)=enum."$GPGGA"
  in  "GNSS Serial cfg":T9={"Port"="COM10", "rate"=115200}
  in  "GNSS Serial delay":u32=20
  out "Raw NMEA":string
  out "Serial bufferN":u32(graph)
  in  "Local Time offset":u32=9
  in  "Send-Serial config":T10={"NMEA out port"="", "baud rate"=9600}
  in  "Data w sel":bool
  in  "Send Serial delay ms":u32=900
  out "log path":string
  out "TM array":cluster{"Y(E)":dbl, "X(N)":dbl}[](array[cluster])
  out "error out":errorcluster
  out "Mount point arr":string[](array[string])
  in  "Ntrip accounts DB index":u32(slide) scale=0.0..9.0
  in  "Ntrip accounts DB":T11[](array[typedef])
  in  "update mount point":bool
  in  "Select Mount points":u16(ring) items=["SONP-RTCM32", "GANS-RTCM32", "GUMC-RTCM32", "DBON-RTCM32", "YONS-RTCM23", "SONP-RTCM23", "GUMC-RTCM23", "GANS-RTCM31", "YONS-CMRx", "SONP-RTCM31", "GUMC-RTCM31", "GANS-RTCM23", "DBON-RTCM23", "DBON-RTCM31", "YONS-RTCM31", "YONS-RTCM32-M5", "VRS-RTCM32-M5", "VRS-RTCM31", "VRS-CMRx", "VRS-CMRplus"]
  out "RTCM recv":string
  in  "Ntrip connect":bool
  out "SourceTable recv-str":string
  out "RTCM arr":u8[](array[numeric]) format="%02x"
  in  "Current Ntrip account":T11={"address"="gnss.eseoul.go.kr", "port "=2101, "id"="seoul", "pwd"="seoul", "ref pt"="YONS-RTCM32-M5"}
  # "GNSS/GPS Test Program"
  # "Made by ybbaek https://github.com/yunbum"
  # "Build ver: 1.0"
  # "RL Connect"
  # "Network Settings"
  # "Commands"
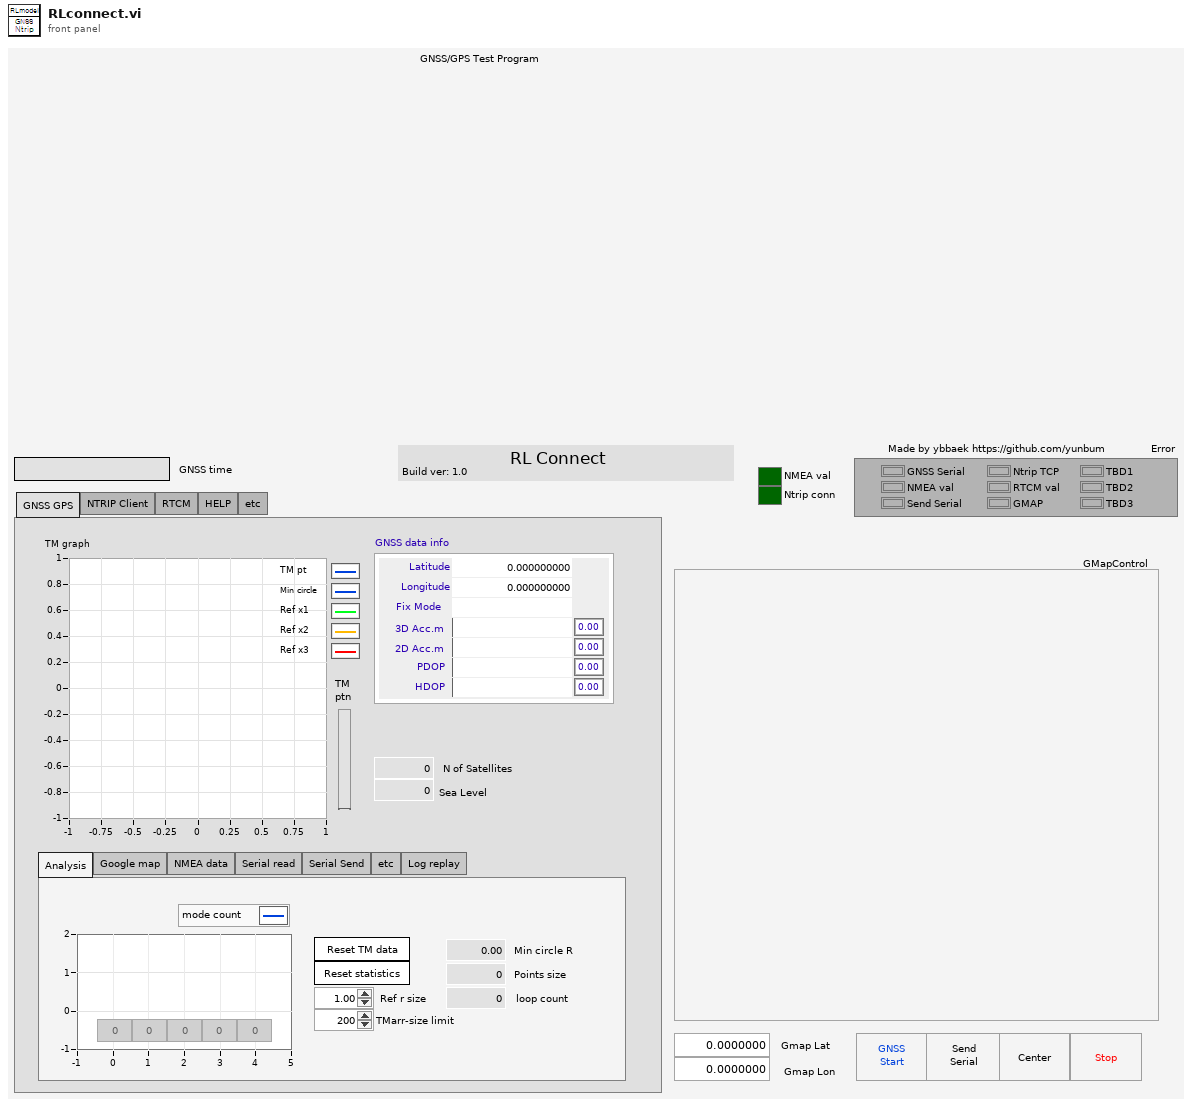
[diagram p1: front panel]
types:
  T1 = typedef "Ntrip error-leds.ctl" = cluster{"GNSS Serial":u8, "NMEA val":u8, "Send Serial":u8, "Ntrip TCP":u8, "RTCM val":u8, "GMAP":u8, "TBD1":u8, "TBD2":u8, "TBD3":u8}
  T2 = enum32{"GNSS GPS", "NTRIP Client", "RTCM", "HELP", "etc"}
  T3 = cluster{"TM array":cluster{"Y(E)":dbl, "X(N)":dbl}[]}[]
  T4 = typedef "ublox-ui_main.ctl" = cluster{"Latitude":dbl, "Longitude":dbl, "Fix Mode":string, "3D Acc.m":dbl, "2D Acc.m":dbl, "PDOP":dbl, "HDOP":dbl}
  T5 = enum32{"Analysis", "Google map", "NMEA data", "Serial read", "Serial Send", "etc", "Log replay"}
  T6 = enum16{"none", "arrow", "blue", "blue_small", "blue_dot", "blue_pushpin", "brown_small", "gray_small", "green", "green_small", "green_dot", "green_pushpin", "green_big_go", "yellow", "yellow_small", "yellow_dot", "yellow_big_pause", "yellow_pushpin", "lightblue", "lightblue_dot", "lightblue_pushpin", "orange", "orange_small", "orange_dot", "pink", "pink_dot", "pink_pushpin", "purple", "purple_small", "purple_dot", "purple_pushpin", "red", "red_small", "red_dot", "red_pushpin", "red_big_stop", "black_small", "white_small"}
  T7 = cluster{"GxGGA":string, "GxGSV":string, "GNRMC":string, "GxTXT":string, "GxGSA":string, "GxGLL":string}
  T8 = enum16{"$GPGSV", "$GLGSV", "$GPGGA", "$GAGSV", "$GBGSV", "$GNGLL", "$GNGGA", "$GNGSA", "$GNRMC", "$GNVTG"}
  T9 = typedef "gnss_config-2.ctl" = cluster{"Port":refnum<visa-resource-name>, "rate":u32}
  T10 = cluster{"NMEA out port":refnum<visa-resource-name>, "baud rate":u32}
  T11 = typedef "Ntrip_Account_db.ctl" = cluster{"address":string, "port ":u16, "id":string, "pwd":string, "ref pt":string}
  T12 = enum16{"Config Save", "Config Load", "LastRUN Save", "LastRUN Load"}
  T13 = typedef "cmd_common.ctl" = enum16{"read", "write"}
  T14 = typedef "cmd_ini-RW.ctl" = enum16{"ini", "read", "write"}
  T15 = typedef "cmd_ini-add-read.ctl" = enum16{"ini", "add", "read"}
  T16 = typedef "GNSS-Ntrip ref.ctl" = cluster{"Mount point arr":refnum<vi>, "Select Mount points":refnum<vi>}
  T17 = enum8{"Enabled", "Disabled", "Disabled and Grayed Out"}
  T18 = typedef "GNSS-Ntrip config.ctl" = cluster{"Ntrip accounts DB":T11[], "Mount points":u16, "Ref r size":dbl, "TMarr limit":i32, "Sel NMEA type":enum16{"$GPGSV", "$GLGSV", "$GPGGA", "$GAGSV", "$GBGSV", "$GNGLL", "$GNGGA", "$GNGSA", "$GNRMC", "$GNVTG"}, "Local Time offset":u32, "GNSS Serial delay":u32, "Send Serial delay":u32, "Send Serial config":cluster{"NMEA out port":refnum<visa-resource-name>, "baud rate":u32}, "Mount point arr":string[], "Ntrip account DB index":u32}
  T19 = cluster{"Gmap Lat":refnum<vi>, "Gmap Lon":refnum<vi>, "Lat Dbclk":refnum<vi>, "Lon Dbclk":refnum<vi>, "zoom":refnum<vi>, "PinDropMrkr":refnum<vi>}
  T20 = typedef "GNSS-Ntrip process val.ctl" = cluster{"GNSS time":string, "Ntrip conn":bool, "NMEA val":bool, "ycenter_TM":dbl, "xcenter_TM":dbl, "TM ref circles":cluster{"Y(E)":dbl, "X(N)":dbl}[], "RTCM recv-str":string, "GNSS Serail buff N":u32, "Sel NMEA type":enum16{"$GPGSV", "$GLGSV", "$GPGGA", "$GAGSV", "$GBGSV", "$GNGLL", "$GNGGA", "$GNGSA", "$GNRMC", "$GNVTG"}, "RTCM recv_sourcetable":string, "NMEA cluster":cluster{"GxGGA":string, "GxGSV":string, "GNRMC":string, "GxTXT":string, "GxGSA":string, "GxGLL":string}, "Sel NMEA str":string, "NMEA recv-str":string}
  T21 = typedef "gmap_fgv-cmd.ctl" = enum16{"marker type change", "save_image", "coll of points", "zoom n center markers", "add overlay reference", "read", "zoom", "set position by keyword", "set map provider", "map provider update", "create", "add marker", "clear marker", "close"}
  T22 = typedef "error_state-val.ctl" = enum16{"na", "error", "OK"}
  T23 = typedef "NMEA.lvlib/NMEA_LatitudeDirection.ctl" = enum16{"", "North", "South"}
  T24 = typedef "NMEA.lvlib/NMEA_LongitudeDirection.ctl" = enum16{"", "East", "West"}
  T25 = typedef "NMEA.lvlib/NMEA_GPS-Quality.ctl" = enum16{"Invalid", "GPS fix (SPS)", "DGPS fix", "PPS fix", "Real Time Kinematic", "Float RTK", "estimated", "Manual input mode", "Simulation mode"}
  T26 = cluster{"$GPGGA-message_OUT":cluster{"TimeStamp":timestamp, "Latitude":dbl, "Latitude-Direction":T23, "Longitude":dbl, "Longitude-Direction":T24, "GPS-Quality":T25, "N of Satellites":i32, "HDOP":dbl, "Altitude above Mean-Sea-Level":dbl, "Geoidal separation":dbl, "Time since last DGPS update":dbl, "DGPS reference station ID":i32}}
  T27 = cluster{"NA":u32, "valid":u32, "DGPS":u32, "RTK float":u32, "RTK fixed":u32}
  T28 = cluster{"TM array":cluster{"Y(E)":dbl, "X(N)":dbl}[]}
  T29 = cluster{"Ntrip tcp":bool, "GNSS serial":bool, "RTCM serial":bool, "Send serial":bool}
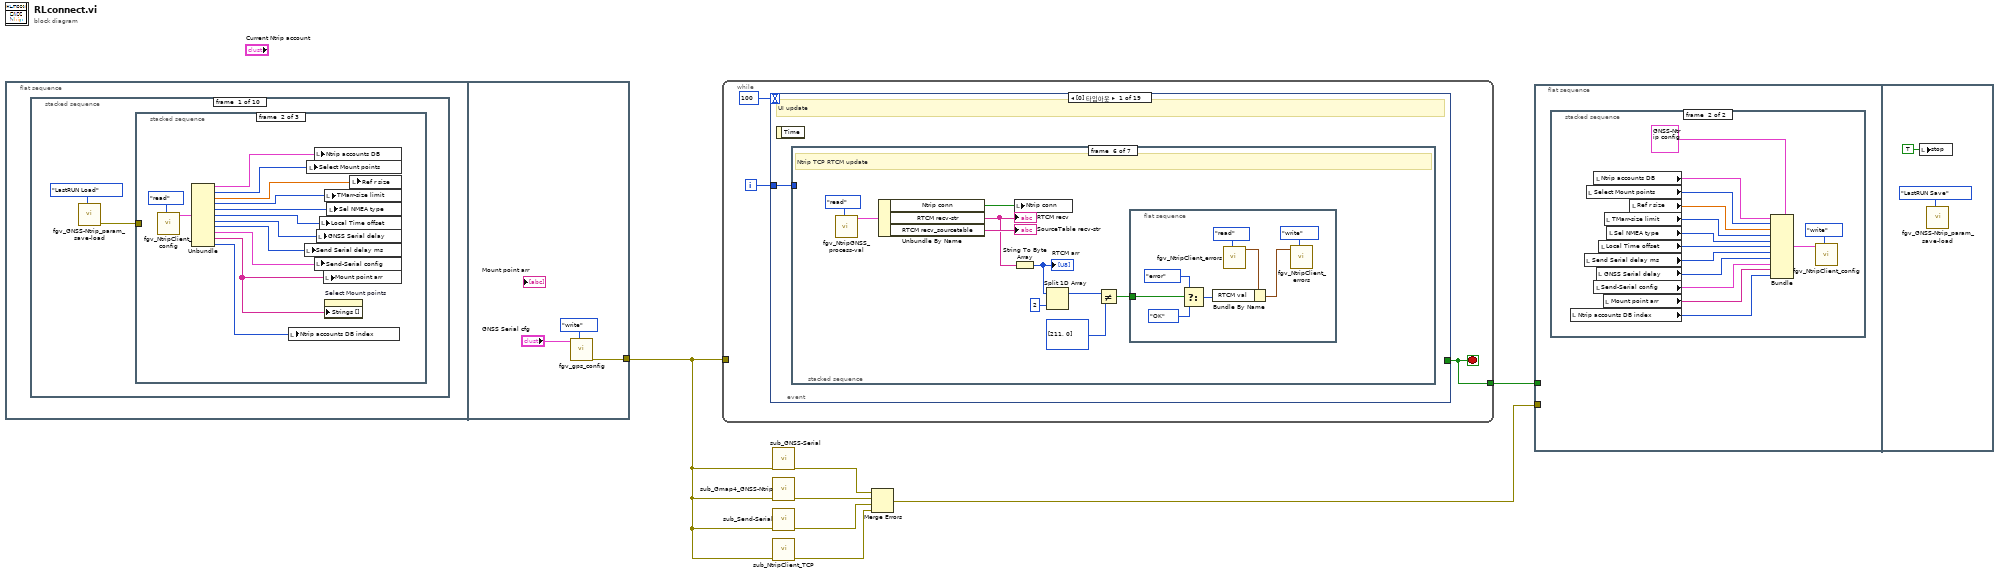
[diagram p0: block diagram]
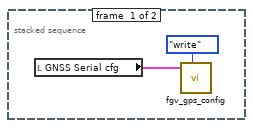
[diagram p2: hidden frame]
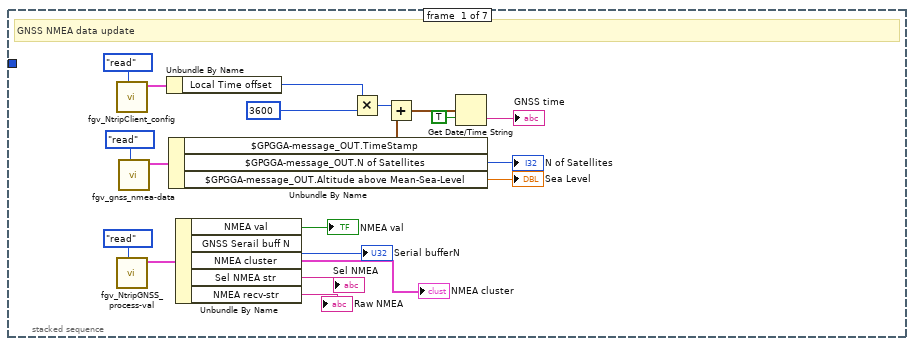
[diagram p3: hidden frame]
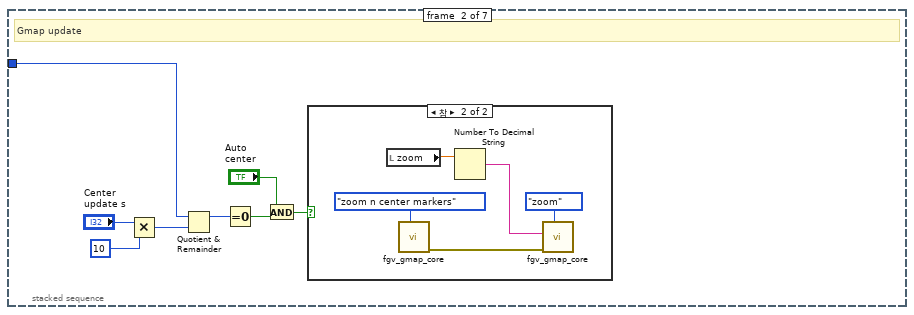
[diagram p4: hidden frame]
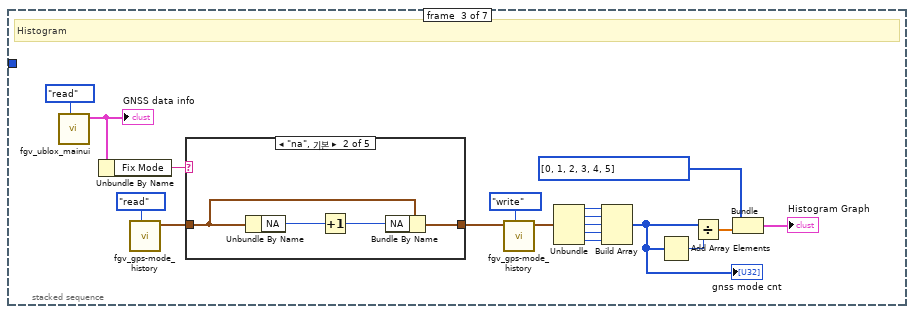
[diagram p6: hidden frame]
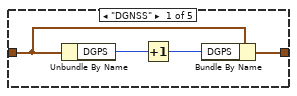
[diagram p7: hidden frame]
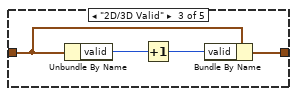
[diagram p8: hidden frame]
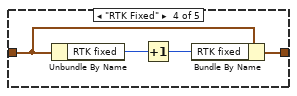
[diagram p9: hidden frame]
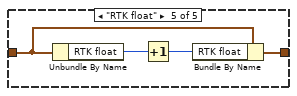
[diagram p10: hidden frame]
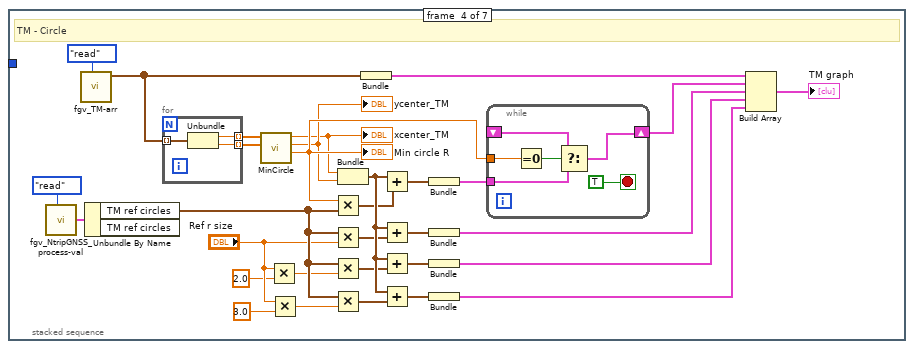
[diagram p11: hidden frame]
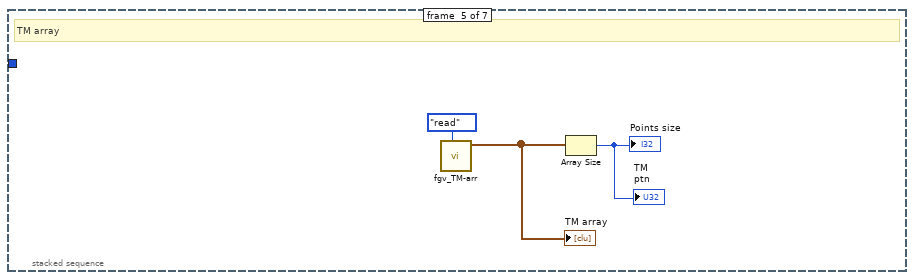
[diagram p12: hidden frame]
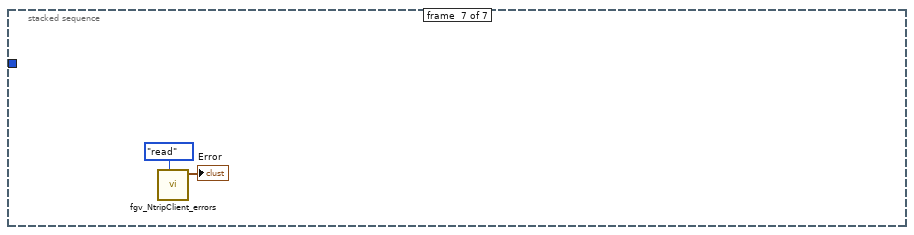
[diagram p13: hidden frame]
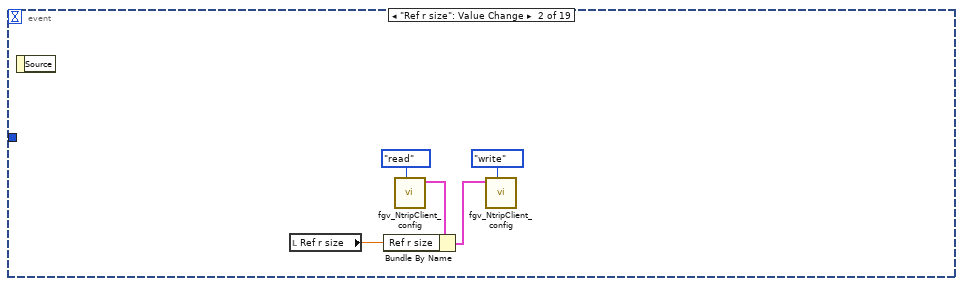
[diagram p14: hidden frame]
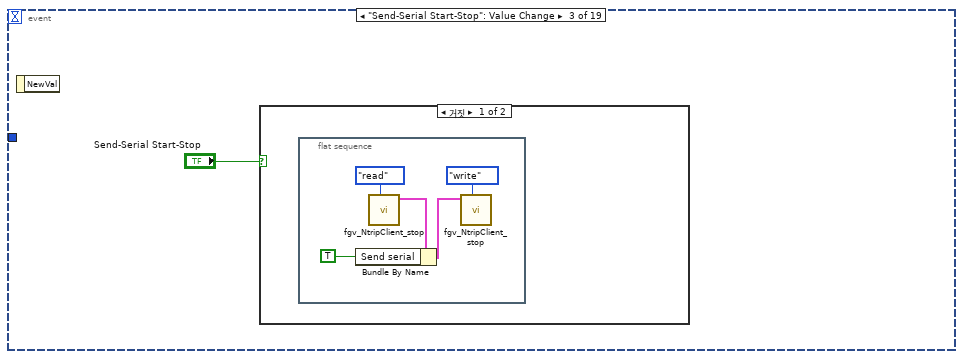
[diagram p15: hidden frame]
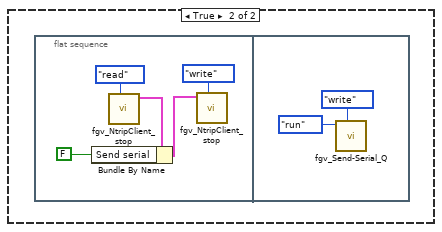
[diagram p16: hidden frame]
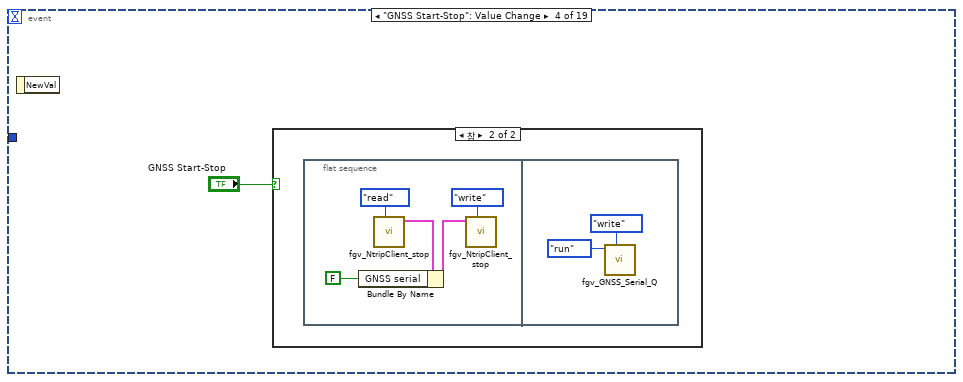
[diagram p17: hidden frame]
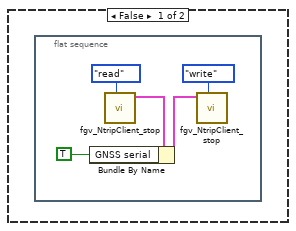
[diagram p18: hidden frame]
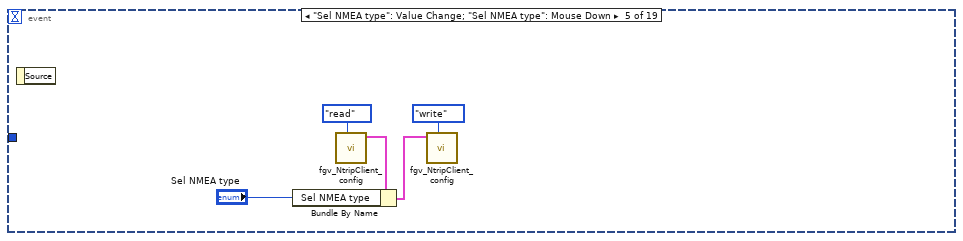
[diagram p19: hidden frame]
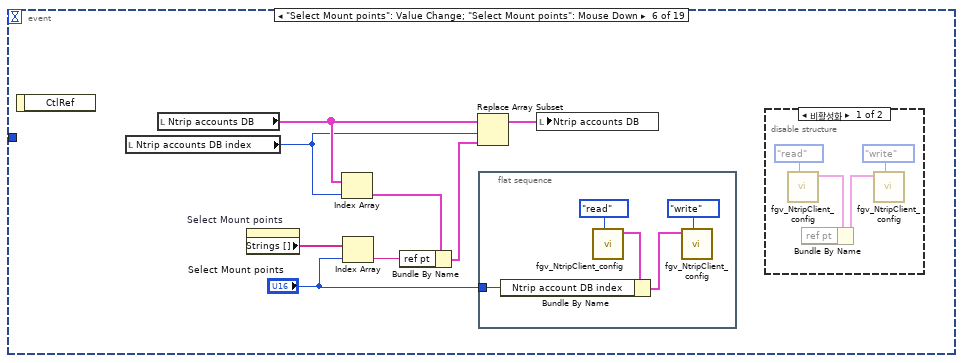
[diagram p20: hidden frame]
diagram:
  n1 = flat-sequence {
    tunnel: [w78] -> w6
    frame #0 {
      n2 = stacked-sequence {
        frame #0 {
          n3 = call "fgv_GNSS-Ntrip_param_save-load.vi"("ctl"=T12."LastRUN Load") -> ("error out"=w8:errorcluster)  [unwired: 9 in, 1 out]
          n4 = stacked-sequence {
            tunnel: w8 -> [_ _ _]
            frame #0 {
              n5 = call "fgv_gps_config.vi"("cmd"=enum16{"read", "write"}."read") -> ("GNSS cfg out"=w10:T9)  [unwired: 9 in, 1 out]
              n6 = local write "GNSS Serial cfg"(w10) -> ()
            }
            frame #1 {
              n7 = call "fgv_NtripClient_config.vi"("cmd"=cmd_common."read") -> ("config val out"=w23:T18)  [unwired: 10 in]
              n8 = Unbundle(w23) -> ("Ntrip accounts DB"=w21:T11[], "Mount points"=w20:u16, "Ref r size"=w19:dbl, "TMarr limit"=w18:i32, "Sel NMEA type"=w15:T8, "Local Time offset"=w14:u32, "GNSS Serial delay"=w13:u32, "Send Serial delay"=w22:u32, "Send Serial config"=w16:T10, "Mount point arr"=w17:string[], "Ntrip account DB index"=w12:u32)
              n9 = local write "Ntrip accounts DB index"(w12) -> ()
              n10 = local write "Send Serial delay ms"(w22) -> ()
              n11 = local write "Select Mount points"(w20) -> ()
              n12 = local write "Ntrip accounts DB"(w21) -> ()
              n13 = local write "Send-Serial config"(w16) -> ()
              n14 = local write "GNSS Serial delay"(w13) -> ()
              n15 = local write "Local Time offset"(w14) -> ()
              n16 = local write "Mount point arr"(w17) -> ()
              n17 = local write "TMarr-size limit"(w18) -> ()
              n18 = property on="Select Mount points" class="Ring (엄격한)"("Strings []"=w17) -> ()  [unwired: 2 in, 2 out]
              n19 = local write "Sel NMEA type"(w15) -> ()
              n20 = local write "Ref r size"(w19) -> ()
            }
            frame #2 {
            }
          }
        }
        frame #1 {
          n21 = call "fgv_gps-mode_history.vi"("cmd"=cmd_ini-RW."ini") -> ()  [unwired: 10 in, 1 out]
          n22 = call "fgv_RTCM_TCP_Q.vi"("cmd"=enum16{"create", "write", "read", "close"}."create") -> ()  [unwired: 9 in, 2 out]
          n23 = call "fgv_global-stop.vi"("cmd"=enum16{"init", "stop", "read"}."init") -> ()  [unwired: 10 in, 1 out]
          n24 = call "fgv_Send-Serial_Q.vi"("cmd"=enum16{"create", "write", "read", "close"}."create") -> ()  [unwired: 9 in, 2 out]
          n25 = call "fgv_TM-arr.vi"("cmd"=cmd_ini-add-read."ini") -> ()  [unwired: 10 in, 1 out]
          n26 = call "fgv_GNSS_Serial_Q.vi"("cmd"=enum16{"create", "write", "read", "close"}."create") -> ()  [unwired: 9 in, 2 out]
          n27 = call "fgv_NtripGNSS_process-val.vi"("cmd"=cmd_ini-RW."ini") -> ()  [unwired: 10 in, 1 out]
          n28 = call "fgv_NtripClient_stop.vi"("cmd"=cmd_ini-RW."ini") -> ()  [unwired: 10 in, 1 out]
          n29 = call "fgv_NtripClient_errors.vi"("cmd"=enum16{"init", "read", "write"}."init") -> ()  [unwired: 9 in, 2 out]
        }
        frame #2 {
          n30 = control-ref of="zoom"() -> (w45:refnum<vi>)
          n31 = control-ref of="Gmap Lat"() -> (w41:refnum<vi>)
          n32 = control-ref of="Gmap Lon"() -> (w42:refnum<vi>)
          n33 = control-ref of="Lat Dbclk"() -> (w43:refnum<vi>)
          n34 = control-ref of="Lon Dbclk"() -> (w44:refnum<vi>)
          n35 = control-ref of="PinDropMrkr"() -> (w46:refnum<vi>)
          n36 = control-ref of="Mount point arr"() -> (w38:refnum<vi>)
          n37 = control-ref of="Select Mount points"() -> (w35:refnum<vi>)
          n38 = Bundle("Gmap Lat"=w41, "Gmap Lon"=w42, "Lat Dbclk"=w43, "Lon Dbclk"=w44, "zoom"=w45, "PinDropMrkr"=w46) -> (w47:T19)  [unwired: 1 in]
          n39 = Bundle(cluster=T16 {"Mount point arr"=refnum, "Select Mount points"=refnum} ("ref 2"), "Mount point arr"=w38, "Select Mount points"=w35) -> (w36:T16)
          n40 = call "fgv_ctr-ref_gmap.vi"("cmd"=cmd_common."write", "ref in"=w47) -> ()  [unwired: 9 in, 1 out]
          n41 = call "fgv_ctrl-ref_cluster.vi"("cmd"=enum16{"read", "write"}."write", "ref"=w47) -> ()  [unwired: 9 in, 1 out]
          n42 = call "fgv_GNSS-Ntrip_ctrl-refs.vi"("cmd"=cmd_common."write", "ref"=w36) -> ()  [unwired: 9 in, 1 out]
        }
        frame #3 {
          n43 = call "fgv_NtripClient_config.vi"("cmd"=cmd_common."read") -> ("config val out"=w52:T18)  [unwired: 10 in]
          n44 = Bundle By Name(cluster=w52, "Send Serial config"="Send-Serial config") -> (w51:T18)
          n45 = call "fgv_NtripClient_config.vi"("cmd"=cmd_common."write", "config val"=w51) -> ()  [unwired: 9 in, 1 out]
        }
        frame #4 {
          n46 = call "sub_gmap_init.vi"("GMapControl"="GMapControl") -> ()  [unwired: 10 in, 1 out]
        }
        frame #5 {
          n47 = call "sub_log_fine-name.vi"() -> ("log path"=→"log path":string)  [unwired: 11 in]
        }
        frame #6 {
          w56 = 100
          n48 = Increment(x=w56) -> (x+1=w63:i32)
          n49 = Divide(x=6.283185307179586, y=w56) -> (x/y=w62:dbl)
          n50 = for {
            N: w63 -> [_]
            tunnel: w62 -> [w68]
            tunnel: [w64] -> w59 mode=indexing
            i -> [w69]
            n51 = Multiply(x=w68, y=w69) -> (x*y=w67:dbl)
            n52 = Sine & Cosine(0:w67) -> (1:w66:dbl, 2:w65:dbl)
            n53 = Bundle(w66, w65) -> (w64:cluster{dbl, dbl})  [unwired: 1 in]
          }
          n54 = call "fgv_NtripGNSS_process-val.vi"("cmd"=cmd_ini-RW."read") -> ("process val out"=w61:T20)  [unwired: 10 in]
          n55 = Bundle By Name(cluster=w61, "TM ref circles"=w59) -> (w60:T20)
          n56 = call "fgv_NtripGNSS_process-val.vi"("cmd"=cmd_ini-RW."write", "process val"=w60) -> ()  [unwired: 9 in, 1 out]
        }
        frame #7 {
          (unwired) "ICY 200 OK" ("정규식")
          w70 = "" ("read raw")
          w72 = FALSE ("정지")
          n57 = disable-structure shown="비활성화" {
            frame Disabled {
              n58 = local write "Ntrip accounts DB index"(u32 0 ("Ntrip accounts DB index")) -> ()
            }
            frame Enabled {
            }
          }
          n59 = local write "Raw NMEA"(w70) -> ()
          n60 = local write "Sel NMEA"(w70) -> ()
          n61 = local write "RTCM recv"(w70) -> ()
          n62 = local write "SourceTable recv-str"(w70) -> ()
          n63 = local write "stop"(w72) -> ()
          n64 = local write "GNSS Start-Stop"(w72) -> ()
          n65 = local write "Send-Serial Start-Stop"(w72) -> ()
          n66 = local write "Ntrip connect"(w72) -> ()
          "Ntrip conn" <- FALSE ("ntrip val")
          "error out" <- errorcluster {"status"=FALSE, "code"=0, "source"=""} ("error out")
        }
        frame #8 {
          n67 = property on="TM\nptn" class="Slide (엄격한)"("Scale.Marker.Selection End"="TMarr-size limit") -> ()  [unwired: 2 in, 2 out]
          n68 = property on="Select Mount points" class="Ring (엄격한)"("DisabledEnum"=T17."Enabled" ("비활성화")) -> ()  [unwired: 2 in, 2 out]
        }
        frame #9 {
        }
      }
    }
    frame #1 {
      n69 = call "fgv_gps_config.vi"("cmd"=enum16{"read", "write"}."write", "GNSS cfg"="GNSS Serial cfg") -> ("error out"=w78:errorcluster)  [unwired: 8 in, 1 out]
    }
  }
  n70 = while {
    tunnel: w6 -> [_]
    tunnel: [w82] -> w7
    i -> [w80]
    stop <- w82 stop-if-true
    n71 = event shown="[0] 타임아웃" {
      selector: _ -> [_ _ _ _ _ _ _ _ _ _ _ _ _ _ _ _ _ _ _]
      dyn-events: _ -> [_ _ _ _ _ _ _ _ _ _ _ _ _ _ _ _ _ _ _]
      timeout: 100 -> [_ _ _ _ _ _ _ _ _ _ _ _ _ _ _ _ _ _ _]
      tunnel: [_ _ _ _ _ _ _ _ _ _ w296 _ _ _ _ _ _ _ _] -> w82
      tunnel: w80 -> [w83 _ _ _ _ _ _ _ _ _ _ _ _ _ _ _ _ _ _]
      event Timeout {
        # "UI update"
        n72 = event-data() -> ()  [unwired: 1 in, 1 out]
        n73 = stacked-sequence {
          tunnel: w83 -> [_ w104 _ _ _ _ _]
          frame #0 {
            # "GNSS NMEA data update"
            n74 = call "fgv_NtripClient_config.vi"("cmd"=cmd_common."read") -> ("config val out"=w96:T18)  [unwired: 10 in]
            n75 = call "fgv_NtripGNSS_process-val.vi"("cmd"=cmd_ini-RW."read") -> ("process val out"=w87:T20)  [unwired: 10 in]
            n76 = call "fgv_gnss_nmea-data.vi"("cmd"=cmd_common."read") -> ("nmea-data out"=w101:T26)  [unwired: 10 in]
            n77 = Unbundle By Name(w96) -> ("Local Time offset"=w95:u32)
            n78 = Unbundle By Name(w101) -> ("$GPGGA-message_OUT.TimeStamp"=w100:timestamp, "$GPGGA-message_OUT.N of Satellites"=→"N of Satellites":i32, "$GPGGA-message_OUT.Altitude above Mean-Sea-Level"=→"Sea Level":dbl)
            n79 = Unbundle By Name(w87) -> ("NMEA val"=→"NMEA val":bool, "GNSS Serail buff N"=→"Serial bufferN":u32, "NMEA cluster"=→"NMEA cluster":T7, "Sel NMEA str"=→"Sel NMEA":string, "NMEA recv-str"=→"Raw NMEA":string)
            n80 = Multiply(x=w95, y=u32 3600) -> (x*y=w103:u32)
            n81 = Add(x=w103, y=w100) -> (x+y=w102:timestamp)
            n82 = Get Date/Time String(seconds (now)=w102, want seconds? (F)=TRUE ("초 보이기? (거짓)")) -> (time string=→"GNSS time":string)  [unwired: 1 in, 1 out]
          }
          frame #1 {
            # "Gmap update"
            n83 = Multiply(x="Center \nupdate s", y=10) -> (x*y=w105:i32)
            n84 = Quotient & Remainder(x=w104, y=w105) -> (x-y*floor(x/y)=w109:i32)  [unwired: 1 out]
            n85 = Equal To 0?(x=w109) -> (x = 0?=w110:bool)
            n86 = And(x="Auto\ncenter", y=w110) -> (x .and. y?=w111:bool)
            n87 = case shown="참" w111 {
              frame False {
              }
              frame True {
                n88 = local read "zoom"() -> (w116:dbl)
                n89 = call "fgv_gmap_core.vi"("cmd"=gmap_fgv-cmd."zoom n center markers") -> ("error out"=w112:errorcluster)  [unwired: 7 in, 3 out]
                n90 = Number To Decimal String(number=w116) -> (decimal integer string=w115:string)  [unwired: 1 in]
                n91 = call "fgv_gmap_core.vi"(7:"cmd"=gmap_fgv-cmd."zoom" ("cmd"), "error in"=w112, 10:"cmd"=w115) -> ()  [unwired: 5 in, 4 out]
              }
            }
          }
          frame #2 {
            # "Histogram"
            n92 = call "fgv_ublox_mainui.vi"("cmd"=cmd_common."read") -> ("MainUI gnss out"=w121:T4)  [unwired: 10 in]
            "GNSS data info" <- w121
            n93 = Unbundle By Name(w121) -> ("Fix Mode"=w122:string)
            n94 = call "fgv_gps-mode_history.vi"("cmd"=cmd_ini-RW."read") -> ("data out"=w123:T27)  [unwired: 10 in]
            n95 = case shown="\"na\", 기본" w122 {
              tunnel: w123 -> [w138 w142 w146 w150 w154]
              tunnel: [w137 w141 w145 w149 w153] -> w124
              frame "DGNSS" {
                n96 = Unbundle By Name(w138) -> ("DGPS"=w136:u32)
                n97 = Increment(x=w136) -> (x+1=w135:u32)
                n98 = Bundle By Name(cluster=w138, "DGPS"=w135) -> (w137:T27)
              }
              frame "na", Default {
                n99 = Unbundle By Name(w142) -> ("NA"=w140:u32)
                n100 = Increment(x=w140) -> (x+1=w139:u32)
                n101 = Bundle By Name(cluster=w142, "NA"=w139) -> (w141:T27)
              }
              frame "2D/3D Valid" {
                n102 = Unbundle By Name(w146) -> ("valid"=w144:u32)
                n103 = Increment(x=w144) -> (x+1=w143:u32)
                n104 = Bundle By Name(cluster=w146, "valid"=w143) -> (w145:T27)
              }
              frame "RTK Fixed" {
                n105 = Unbundle By Name(w150) -> ("RTK fixed"=w148:u32)
                n106 = Increment(x=w148) -> (x+1=w147:u32)
                n107 = Bundle By Name(cluster=w150, "RTK fixed"=w147) -> (w149:T27)
              }
              frame "RTK float" {
                n108 = Unbundle By Name(w154) -> ("RTK float"=w152:u32)
                n109 = Increment(x=w152) -> (x+1=w151:u32)
                n110 = Bundle By Name(cluster=w154, "RTK float"=w151) -> (w153:T27)
              }
            }
            n111 = call "fgv_gps-mode_history.vi"("cmd"=cmd_ini-RW."write", "data"=w124) -> ("data out"=w125:T27)  [unwired: 9 in]
            n112 = Unbundle(w125) -> ("NA"=w126:u32, "valid"=w130:u32, "DGPS"=w129:u32, "RTK float"=w128:u32, "RTK fixed"=w127:u32)
            n113 = Build Array(w126, w130, w129, w128, w127) -> (w134:u32[])
            "gnss mode cnt" <- w134
            n114 = Add Array Elements(numeric array=w134) -> (sum=w132:u32)
            n115 = Divide(x=w134, y=w132) -> (x/y=w133:dbl[])
            n116 = Bundle(i32[] [0, 1, 2, 3, 4, 5], w133) -> (→"Histogram Graph":cluster{i32[], dbl[]})  [unwired: 1 in]
          }
          frame #3 {
            # "TM - Circle"
            n117 = call "fgv_NtripGNSS_process-val.vi"("cmd"=cmd_ini-RW."read") -> ("process val out"=w183:T20)  [unwired: 10 in]
            n118 = call "fgv_TM-arr.vi"("cmd"=cmd_ini-add-read."read") -> ("TM array"=w185:cluster{"Y(E)":dbl, "X(N)":dbl}[])  [unwired: 10 in]
            n119 = Unbundle By Name(w183) -> ("TM ref circles"=w184:cluster{"Y(E)":dbl, "X(N)":dbl}[])  [unwired: 1 out]
            n120 = for {
              tunnel: [w194] -> w160 mode=indexing
              tunnel: [w193] -> w161 mode=indexing
              tunnel: w185 -> [w192] mode=indexing
              n121 = Unbundle(w192) -> ("Y(E)"=w194:dbl, "X(N)"=w193:dbl)
            }
            n122 = call "MinCircle.vi"("y"=w161, "x"=w160) -> ("r"=w170:dbl, "yc"=w163:dbl, "xc"=w162:dbl)  [unwired: 6 in, 1 out]
            "xcenter_TM" <- w162
            "ycenter_TM" <- w163
            "Min circle R" <- w170
            n123 = Multiply(x="Ref r size", y=2.0) -> (x*y=w175:dbl)
            n124 = Multiply(x="Ref r size", y=3.0) -> (x*y=w156:dbl)
            n125 = Multiply(x=w170, y=w184) -> (x*y=w164:cluster{"Y(E)":dbl, "X(N)":dbl}[])
            n126 = Multiply(x=w184, y="Ref r size") -> (x*y=w174:cluster{"Y(E)":dbl, "X(N)":dbl}[])
            n127 = Multiply(x=w184, y=w175) -> (x*y=w173:cluster{"Y(E)":dbl, "X(N)":dbl}[])
            n128 = Multiply(x=w184, y=w156) -> (x*y=w176:cluster{"Y(E)":dbl, "X(N)":dbl}[])
            n129 = Bundle("xc"=w162, "yc"=w163) -> (w177:cluster{"xc":dbl, "yc":dbl})  [unwired: 1 in]
            n130 = Bundle("TM array"=w185) -> (w166:T28)  [unwired: 1 in]
            n131 = Add(x=w177, y=w164) -> (x+y=w165:cluster{dbl, dbl}[])
            n132 = Add(x=w177, y=w174) -> (x+y=w171:cluster{dbl, dbl}[])
            n133 = Add(x=w177, y=w173) -> (x+y=w179:cluster{dbl, dbl}[])
            n134 = Add(x=w177, y=w176) -> (x+y=w178:cluster{dbl, dbl}[])
            n135 = Bundle(w165) -> (w168:cluster{cluster{dbl, dbl}[]})  [unwired: 1 in]
            n136 = Bundle(w171) -> (w172:cluster{cluster{dbl, dbl}[]})  [unwired: 1 in]
            n137 = Bundle(w179) -> (w180:cluster{cluster{dbl, dbl}[]})  [unwired: 1 in]
            n138 = Bundle(w178) -> (w181:cluster{cluster{dbl, dbl}[]})  [unwired: 1 in]
            n139 = while {
              shift-right: [w186] -> w169
              shift-left: _ -> [w188]
              tunnel: w170 -> [w190]
              tunnel: w168 -> [w187]
              stop <- TRUE stop-if-true
              n140 = Equal To 0?(x=w190) -> (x = 0?=w189:bool)
              n141 = Select(t=w188, s=w189, f=w187) -> (s? t:f=w186:cluster{cluster{dbl, dbl}[]})
            }
            n142 = Build Array(w166, w169, w172, w180, w181) -> (→"TM graph":T3)
          }
          frame #4 {
            # "TM array"
            n143 = call "fgv_TM-arr.vi"("cmd"=cmd_ini-add-read."read") -> ("TM array"=w195:cluster{"Y(E)":dbl, "X(N)":dbl}[])  [unwired: 10 in]
            "TM array" <- w195
            n144 = Array Size(array=w195) -> (size(s)=→"Points size" →"TM\nptn":i32)
          }
          frame #5 {
            # "Ntrip TCP RTCM update"
            n145 = call "fgv_NtripGNSS_process-val.vi"("cmd"=cmd_ini-RW."read") -> ("process val out"=w204:T20)  [unwired: 10 in]
            n146 = Unbundle By Name(w204) -> ("Ntrip conn"=w205:bool, "RTCM recv-str"=w203:string, "RTCM recv_sourcetable"=→"SourceTable recv-str":string)
            "RTCM recv" <- w203
            n147 = String To Byte Array(string=w203) -> (unsigned byte array=w202:u8[])
            "RTCM arr" <- w202
            n148 = local write "Ntrip conn"(w205) -> ()
            n149 = Split 1D Array(array=w202, index=2 ("인덱스")) -> (first subarray=w200:u8[])  [unwired: 1 out]
            n150 = Not Equal?(x=w200, y=u8[] [211, 0]) -> (x != y?=w198:bool)
            n151 = flat-sequence {
              tunnel: w198 -> [w211]
              frame #0 {
                n152 = Select(t=error_state-val."error", s=w211, f=error_state-val."OK") -> (s? t:f=w208:T22)
                n153 = call "fgv_NtripClient_errors.vi"("cmd"=enum16{"init", "read", "write"}."read") -> ("Error led out"=w213:T1)  [unwired: 9 in, 1 out]
                n154 = Bundle By Name(cluster=w213, "RTCM val"=w208) -> (w212:T1)
                n155 = call "fgv_NtripClient_errors.vi"("cmd"=enum16{"init", "read", "write"}."write", "Error led"=w212) -> ()  [unwired: 8 in, 2 out]
              }
            }
          }
          frame #6 {
            n156 = call "fgv_NtripClient_errors.vi"("cmd"=enum16{"init", "read", "write"}."read") -> ("Error led out"=→"Error":T1)  [unwired: 9 in, 1 out]
          }
        }
      }
      event "Ref r size": Value Change {
        n157 = event-data() -> ()  [unwired: 1 in, 1 out]
        n158 = local read "Ref r size"() -> (w218:dbl)
        n159 = call "fgv_NtripClient_config.vi"("cmd"=cmd_common."read") -> ("config val out"=w222:T18)  [unwired: 10 in]
        n160 = Bundle By Name(cluster=w222, "Ref r size"=w218) -> (w221:T18)
        n161 = call "fgv_NtripClient_config.vi"("cmd"=cmd_common."write", "config val"=w221) -> ()  [unwired: 9 in, 1 out]
      }
      event "Send-Serial Start-Stop": Value Change {
        n162 = event-data() -> ()  [unwired: 1 in, 1 out]
        n163 = case shown="거짓" "Send-Serial Start-Stop" {
          frame False {
            n164 = flat-sequence {
              frame #0 {
                n165 = call "fgv_NtripClient_stop.vi"("cmd"=cmd_ini-RW."read") -> ("local stops out"=w226:T29)  [unwired: 10 in]
                n166 = Bundle By Name(cluster=w226, "Send serial"=TRUE ("Ntrip tcp")) -> (w225:T29)
                n167 = call "fgv_NtripClient_stop.vi"("cmd"=cmd_ini-RW."write", "local stops"=w225) -> ()  [unwired: 9 in, 1 out]
              }
            }
          }
          frame True {
            n168 = flat-sequence {
              frame #0 {
                n169 = call "fgv_NtripClient_stop.vi"("cmd"=cmd_ini-RW."read") -> ("local stops out"=w231:T29)  [unwired: 10 in]
                n170 = Bundle By Name(cluster=w231, "Send serial"=FALSE ("Ntrip tcp")) -> (w230:T29)
                n171 = call "fgv_NtripClient_stop.vi"("cmd"=cmd_ini-RW."write", "local stops"=w230) -> ()  [unwired: 9 in, 1 out]
              }
              frame #1 {
                n172 = call "fgv_Send-Serial_Q.vi"("cmd"=enum16{"create", "write", "read", "close"}."write", "data"=enum16{"run", "check", "stop"}."run") -> ()  [unwired: 8 in, 2 out]
              }
            }
          }
        }
      }
      event "GNSS Start-Stop": Value Change {
        n173 = event-data() -> ()  [unwired: 1 in, 1 out]
        n174 = case shown="참" "GNSS Start-Stop" {
          frame False {
            n175 = flat-sequence {
              frame #0 {
                n176 = call "fgv_NtripClient_stop.vi"("cmd"=cmd_ini-RW."read") -> ("local stops out"=w239:T29)  [unwired: 10 in]
                n177 = Bundle By Name(cluster=w239, "GNSS serial"=TRUE ("Ntrip tcp")) -> (w238:T29)
                n178 = call "fgv_NtripClient_stop.vi"("cmd"=cmd_ini-RW."write", "local stops"=w238) -> ()  [unwired: 9 in, 1 out]
              }
            }
          }
          frame True {
            n179 = flat-sequence {
              frame #0 {
                n180 = call "fgv_NtripClient_stop.vi"("cmd"=cmd_ini-RW."read") -> ("local stops out"=w244:T29)  [unwired: 10 in]
                n181 = Bundle By Name(cluster=w244, "GNSS serial"=FALSE ("Ntrip tcp")) -> (w243:T29)
                n182 = call "fgv_NtripClient_stop.vi"("cmd"=cmd_ini-RW."write", "local stops"=w243) -> ()  [unwired: 9 in, 1 out]
              }
              frame #1 {
                n183 = call "fgv_GNSS_Serial_Q.vi"("cmd"=enum16{"create", "write", "read", "close"}."write", "data"=enum16{"run", "check", "stop"}."run") -> ()  [unwired: 8 in, 2 out]
              }
            }
          }
        }
      }
      event "Sel NMEA type": Value Change; "Sel NMEA type": Mouse Down {
        n184 = event-data() -> ()  [unwired: 1 in, 1 out]
        n185 = call "fgv_NtripClient_config.vi"("cmd"=cmd_common."read") -> ("config val out"=w253:T18)  [unwired: 10 in]
        n186 = Bundle By Name(cluster=w253, "Sel NMEA type"="Sel NMEA type") -> (w252:T18)
        n187 = call "fgv_NtripClient_config.vi"("cmd"=cmd_common."write", "config val"=w252) -> ()  [unwired: 9 in, 1 out]
      }
      event "Select Mount points": Value Change; "Select Mount points": Mouse Down {
        n188 = event-data() -> ()  [unwired: 1 in, 1 out]
        n189 = local read "Ntrip accounts DB index"() -> (w259:u32)
        n190 = local read "Ntrip accounts DB"() -> (w260:T11[])
        n191 = property on="Select Mount points" class="Ring (엄격한)"() -> ("Strings []"=w261:string[])  [unwired: 2 in, 2 out]
        n192 = Index Array(array=w260, index=w259) -> (element=w258:T11)
        n193 = Index Array(array=w261, index="Select Mount points") -> (element=w257:string)
        n194 = Bundle By Name(cluster=w258, "ref pt"=w257) -> (w256:T11)
        n195 = Replace Array Subset(array=w260, new element=w256, index=w259) -> (w255:T11[])
        n196 = flat-sequence {
          tunnel: "Select Mount points" -> [w265]
          frame #0 {
            n197 = call "fgv_NtripClient_config.vi"("cmd"=cmd_common."read") -> ("config val out"=w266:T18)  [unwired: 10 in]
            n198 = Bundle By Name(cluster=w266, "Ntrip account DB index"=w265) -> (w264:T18)
            n199 = call "fgv_NtripClient_config.vi"("cmd"=cmd_common."write", "config val"=w264) -> ()  [unwired: 9 in, 1 out]
          }
        }
        n200 = local write "Ntrip accounts DB"(w255) -> ()
        n201 = disable-structure shown="비활성화" {
          frame Disabled {
            n202 = call "fgv_NtripClient_config.vi"("cmd"=cmd_common."read") -> ("config val out"=w270:T18)  [unwired: 10 in]
            n203 = Bundle By Name(cluster=w270) -> (w269:T18)  [unwired: 1 in]
            n204 = call "fgv_NtripClient_config.vi"("cmd"=cmd_common."write", "config val"=w269) -> ()  [unwired: 9 in, 1 out]
          }
          frame Enabled {
          }
        }
      }
      event "Local Time offset": Value Change {
        n205 = event-data() -> ()  [unwired: 1 in, 1 out]
        n206 = call "fgv_NtripClient_config.vi"("cmd"=cmd_common."read") -> ("config val out"=w273:T18)  [unwired: 10 in]
        n207 = Bundle By Name(cluster=w273, "Local Time offset"="Local Time offset") -> (w271:T18)
        n208 = call "fgv_NtripClient_config.vi"("cmd"=cmd_common."write", "config val"=w271) -> ()  [unwired: 9 in, 1 out]
      }
      event "Ntrip accounts DB index": Value Change; "Ntrip accounts DB index": Mouse Down {
        n209 = event-data() -> ()  [unwired: 1 in, 1 out]
        n210 = Build Array("Ntrip accounts DB index") -> (w282:u32[])
        n211 = property on="Ntrip accounts DB" class="Arr (엄격한)"("Index Values"=w282) -> ()  [unwired: 2 in, 2 out]
        n212 = call "fgv_NtripClient_config.vi"("cmd"=cmd_common."read") -> ("config val out"=w281:T18)  [unwired: 10 in]
        n213 = Bundle By Name(cluster=w281, "Ntrip accounts DB"="Ntrip accounts DB", "Ntrip account DB index"="Ntrip accounts DB index") -> (w280:T18)
        n214 = call "fgv_NtripClient_config.vi"("cmd"=cmd_common."write", "config val"=w280) -> ()  [unwired: 9 in, 1 out]
      }
      event "GNSS Serial delay": Value Change {
        n215 = event-data() -> ()  [unwired: 1 in, 1 out]
        n216 = call "fgv_NtripClient_config.vi"("cmd"=cmd_common."read") -> ("config val out"=w285:T18)  [unwired: 10 in]
        n217 = Bundle By Name(cluster=w285, "GNSS Serial delay"="GNSS Serial delay") -> (w284:T18)
        n218 = call "fgv_NtripClient_config.vi"("cmd"=cmd_common."write", "config val"=w284) -> ()  [unwired: 9 in, 1 out]
      }
      event "TMarr-size limit": Value Change {
        n219 = event-data() -> ()  [unwired: 1 in, 1 out]
        n220 = local read "TMarr-size limit"() -> (w288:i32)
        n221 = property on="TM\nptn" class="Slide (엄격한)"("Scale.Marker.Selection End"=w288) -> ()  [unwired: 2 in, 2 out]
        n222 = call "fgv_NtripClient_config.vi"("cmd"=cmd_common."read") -> ("config val out"=w292:T18)  [unwired: 10 in]
        n223 = Bundle By Name(cluster=w292, "TMarr limit"=w288) -> (w291:T18)
        n224 = call "fgv_NtripClient_config.vi"("cmd"=cmd_common."write", "config val"=w291) -> ()  [unwired: 9 in, 1 out]
      }
      event "stop": Value Change {
        n225 = event-data() -> ()  [unwired: 1 in, 1 out]
        n226 = call "fgv_GNSS_Serial_Q.vi"("cmd"=enum16{"create", "write", "read", "close"}."close") -> ()  [unwired: 9 in, 2 out]
        n227 = call "fgv_RTCM_TCP_Q.vi"("cmd"=enum16{"create", "write", "read", "close"}."close") -> ()  [unwired: 9 in, 2 out]
        n228 = call "fgv_Send-Serial_Q.vi"("cmd"=enum16{"create", "write", "read", "close"}."close") -> ()  [unwired: 9 in, 2 out]
        n229 = call "fgv_global-stop.vi"("cmd"=enum16{"init", "stop", "read"}."stop") -> ("val_out"=w296:bool)  [unwired: 10 in]
      }
      event "update mount point": Value Change {
        n230 = event-data() -> ()  [unwired: 1 in, 1 out]
        n231 = flat-sequence {
          frame #0 {
          }
          frame #1 {
            n232 = call "fgv_RTCM_TCP_Q.vi"("cmd"=enum16{"create", "write", "read", "close"}."write", "data"=enum16{"run", "check", "stop"}."check") -> ()  [unwired: 8 in, 2 out]
          }
        }
      }
      event "Ntrip accounts DB": Value Change {
        n233 = event-data() -> ()  [unwired: 1 in, 1 out]
        n234 = local read "Ntrip accounts DB"() -> (w300:T11[])
        n235 = call "fgv_NtripClient_config.vi"("cmd"=cmd_common."read") -> ("config val out"=w304:T18)  [unwired: 10 in]
        n236 = Bundle By Name(cluster=w304, "Ntrip accounts DB"=w300) -> (w303:T18)
        n237 = call "fgv_NtripClient_config.vi"("cmd"=cmd_common."write", "config val"=w303) -> ()  [unwired: 9 in, 1 out]
      }
      event "gmap center": Value Change {
        n238 = event-data() -> ()  [unwired: 1 in, 1 out]
        n239 = call "fgv_gmap_core.vi"("cmd"=gmap_fgv-cmd."zoom n center markers") -> ("error out"=w305:errorcluster)  [unwired: 7 in, 3 out]
        n240 = local read "zoom"() -> (w308:dbl)
        n241 = Number To Decimal String(number=w308) -> (decimal integer string=w307:string)  [unwired: 1 in]
        n242 = call "fgv_gmap_core.vi"(7:"cmd"=gmap_fgv-cmd."zoom" ("cmd"), "error in"=w305, 10:"cmd"=w307) -> ()  [unwired: 5 in, 4 out]
      }
      event "Ntrip connect": Value Change {
        n243 = event-data() -> ()  [unwired: 1 in, 1 out]
        n244 = case shown="참" "Ntrip connect" {
          frame False {
            n245 = call "fgv_NtripClient_stop.vi"("cmd"=cmd_ini-RW."read") -> ("local stops out"=w313:T29)  [unwired: 10 in]
            n246 = Bundle By Name(cluster=w313, "Ntrip tcp"=TRUE) -> (w312:T29)
            n247 = call "fgv_NtripClient_stop.vi"("cmd"=cmd_ini-RW."write", "local stops"=w312) -> ()  [unwired: 9 in, 1 out]
          }
          frame True {
            n248 = flat-sequence {
              frame #0 {
                n249 = call "fgv_NtripClient_stop.vi"("cmd"=cmd_ini-RW."read") -> ("local stops out"=w320:T29)  [unwired: 10 in]
                n250 = Bundle By Name(cluster=w320, "Ntrip tcp"=FALSE) -> (w319:T29)
                n251 = call "fgv_NtripClient_stop.vi"("cmd"=cmd_ini-RW."write", "local stops"=w319) -> ()  [unwired: 9 in, 1 out]
              }
              frame #1 {
                n252 = call "fgv_RTCM_TCP_Q.vi"("cmd"=enum16{"create", "write", "read", "close"}."write", "data"=enum16{"run", "check", "stop"}."run") -> ()  [unwired: 8 in, 2 out]
              }
            }
          }
        }
      }
      event "tm data reset": Value Change {
        # "TM GPS data array reset"
        n253 = event-data() -> ()  [unwired: 1 in, 1 out]
        n254 = case shown="참" "tm data reset" {
          frame False {
          }
          frame True {
            n255 = call "fgv_TM-arr.vi"("cmd"=cmd_ini-add-read."ini") -> ()  [unwired: 10 in, 1 out]
          }
        }
      }
      event "zoom": Value Change {
        n256 = event-data() -> ()  [unwired: 1 in, 1 out]
        n257 = local read "zoom"() -> (w326:dbl)
        n258 = Number To Decimal String(number=w326) -> (decimal integer string=w325:string)  [unwired: 1 in]
        n259 = call "fgv_gmap_core.vi"(7:"cmd"=gmap_fgv-cmd."zoom" ("cmd"), 10:"cmd"=w325) -> ()  [unwired: 6 in, 4 out]
      }
      event "gnss mode check": Value Change {
        n260 = event-data() -> ()  [unwired: 1 in, 1 out]
        n261 = call "fgv_gps-mode_history.vi"("cmd"=cmd_ini-RW."ini") -> ()  [unwired: 10 in, 1 out]
      }
      event Value Change {
        n262 = event-data() -> ()  [unwired: 1 in, 1 out]
        n263 = local read "GNSS Serial cfg"() -> (w329:T9)
        n264 = call "fgv_gps_config.vi"("cmd"=enum16{"read", "write"}."write", "GNSS cfg"=w329) -> ()  [unwired: 8 in, 2 out]
      }
    }
  }
  n265 = call "sub_GNSS-Serial.vi"("error in"=w6) -> ("error out"=w2:errorcluster)  [unwired: 10 in]
  n266 = call "sub_Gmap4_GNSS-Ntrip.vi"("error in"=w6) -> ("error out"=w3:errorcluster)  [unwired: 10 in]
  n267 = call "sub_Send-Serial.vi"("error in"=w6) -> ("error out"=w4:errorcluster)  [unwired: 10 in]
  n268 = call "sub_NtripClient_TCP.vi"("error in"=w6) -> ("error out"=w5:errorcluster)  [unwired: 10 in]
  n269 = Merge Errors(w2, w3, w4, w5) -> (w1:errorcluster)
  n270 = flat-sequence {
    tunnel: w7 -> [_]
    tunnel: w1 -> [_]
    frame #0 {
      n271 = stacked-sequence {
        frame #0 {
          n272 = local read "GNSS Serial cfg"() -> (w332:T9)
          n273 = call "fgv_gps_config.vi"("cmd"=enum16{"read", "write"}."write", "GNSS cfg"=w332) -> ()  [unwired: 8 in, 2 out]
        }
        frame #1 {
          n274 = local read "Ntrip accounts DB index"() -> (w333:u32)
          n275 = local read "Send Serial delay ms"() -> (w337:u32)
          n276 = local read "Select Mount points"() -> (w344:u16)
          n277 = local read "Ntrip accounts DB"() -> (w345:T11[])
          n278 = local read "Send-Serial config"() -> (w339:T10)
          n279 = local read "GNSS Serial delay"() -> (w338:u32)
          n280 = local read "Local Time offset"() -> (w336:u32)
          n281 = local read "Mount point arr"() -> (w340:string[])
          n282 = local read "TMarr-size limit"() -> (w342:i32)
          n283 = local read "Sel NMEA type"() -> (w341:T8)
          n284 = local read "Ref r size"() -> (w343:dbl)
          n285 = Bundle(cluster=T18 {"Ntrip accounts DB"=[], "Mount points"=0, "Ref r size"=0.0, "TMarr limit"=0, "Sel NMEA type"=enum."$GPGSV", "Local Time offset"=0, "GNSS Serial delay"=0, "Send Serial delay"=0, "Send Serial config"={"NMEA out port"="", "baud rate"=0}, "Mount point arr"=[], "Ntrip account DB index"=20} ("config val out"), "Ntrip accounts DB"=w345, "Mount points"=w344, "Ref r size"=w343, "TMarr limit"=w342, "Sel NMEA type"=w341, "Local Time offset"=w336, "GNSS Serial delay"=w337, "Send Serial delay"=w338, "Send Serial config"=w339, "Mount point arr"=w340, "Ntrip account DB index"=w333) -> (w334:T18)
          n286 = call "fgv_NtripClient_config.vi"("cmd"=cmd_common."write", "config val"=w334) -> ()  [unwired: 9 in, 1 out]
        }
      }
    }
    frame #1 {
      n287 = local write "stop"(TRUE ("stop")) -> ()
      n288 = call "fgv_GNSS-Ntrip_param_save-load.vi"("ctl"=T12."LastRUN Save") -> ()  [unwired: 9 in, 2 out]
    }
  }
